vi "运维调试_质控单元.vi"() -> ()   [LabVIEW 2016, in "质控单元.lvlib"]
uses:
  <vilib>/Utility/miscctls.llb/LVPointTypeDef.ctl
  <vilib>/Analysis/6fits.llb/Curve Fitting Criteria.ctl
  <vilib>/Plasmionique/MB Master/MB_Master_Serial/MB_Master_Serial.lvclass
  D:/Program Files (x86)/National Instruments/LabVIEW 2016/vi.lib/Plasmionique/MB Master/MB_Master/MB_Master.lvclass
  <vilib>/Utility/config.llb/Read Key (I32).vi
  <vilib>/Utility/config.llb/Read Key (Double).vi
  <vilib>/Utility/config.llb/Read Key (Boolean).vi
  <vilib>/Utility/config.llb/Read Key (U32).vi
  <vilib>/Utility/config.llb/Write Key (I32).vi
  <vilib>/Utility/config.llb/Write Key (Double).vi
  <vilib>/Utility/config.llb/Write Key (Boolean).vi
  <vilib>/Utility/config.llb/Write Key (U32).vi
  <vilib>/Plasmionique/MB Master/MB Master.lvlib
  <vilib>/ptbypt/NI_PtbyPt.lvlib
  <vilib>/Utility/config.llb/NI_LVConfig.lvlib
  <vilib>/Analysis/NI_AALPro.lvlib
panel:
  in  "柱塞泵4":bool
  in  "CODCr量程选择":enum32{"H", "L", "AUTO"}(ring)
  in  "B 4":dbl caption="B4"
  in  "K 4":dbl caption="K4"
  out "通讯指示灯4":bool
  in  "CODCr选择":bool
  out "CODCr传感器故障报警":bool
  out "CODCr超时报警":bool
  out "CODMn超时报警":bool
  out "总磷总氮超时报警":bool
  out "氨氮进样超时报警":bool
  out "CODMn传感器故障报警":bool
  out "总磷总氮传感器故障报警":bool
  out "氨氮传感器故障报警":bool
  in  "CODCr加标回收启动":bool
  in  "CODCr停止":bool
  in  "CODCr排液":bool
  in  "CODCr调试":bool
  out "CODCr加标回收率":dbl caption="加标回收率" format="%.2f"
  out "CODCr加标体积":dbl caption="加标体积" format="%.3f"
  out "CODCr母液浓度":dbl caption="加标母液浓度" format="%.2f"
  out "CODCr加标水杯定容体积":dbl caption="加标水杯定容体积" format="%.2f"
  out "CODCr加标后水样浓度":dbl caption="加标后水样浓度" format="%.2f"
  out "CODCr加标前水样浓度":dbl caption="加标前水样浓度" format="%.2f"
  out "CODCr检出限":dbl caption="检出限" format="%.2f"
  out "CODCr量程":dbl caption="量程" format="%.2f"
  out "CODCr状态":u16(ring) caption="状态" items=["待机", "润洗", "进样", "等待取液", "排液"]
  out "质控流程中":bool
  out "CODMn质控中断报警":bool
  out "总磷质控中断报警":bool
  out "总氮质控中断报警":bool
  out "氨氮质控中断报警":bool
  in  "报警清除":bool
  in  "CODMn量程选择":enum32{"H", "L", "AUTO"}(ring)
  in  "CODMn加标回收启动":bool
  in  "总磷总氮加标回收启动":bool
  in  "氨氮加标回收启动":bool
  in  "总磷量程选择":enum32{"H", "L", "AUTO"}(ring)=enum."AUTO"
  in  "总氮量程选择":enum32{"H", "L", "AUTO"}(ring)=enum."AUTO"
  in  "氨氮量程选择":enum32{"H", "L", "AUTO"}(ring)=enum."AUTO"
  out "线性值":T1
  out "通讯指示灯3":bool
  out "通讯指示灯2":bool
  out "通讯指示灯1":bool
  in  "CODMn选择":bool
  in  "总氮模块选择":bool
  in  "氨氮、总磷模块":bool
  in  "枚举":enum16{"柱塞泵1", "柱塞泵2", "柱塞泵3", "柱塞泵4"}(ring)
  in  "启用":bool
  in  "B 3":dbl caption="B3"
  in  "K 3":dbl caption="K3"
  in  "B 2":dbl caption="B2"
  in  "K 2":dbl caption="K2"
  in  "B":dbl caption="B1"
  in  "K":dbl caption="K1"
  out "r^2":dbl format="%_6g"
  out "拟合方程":string
  in  "实际体积 5":dbl
  in  "标准体积 5":dbl
  in  "实际体积 4":dbl
  in  "标准体积 4":dbl
  in  "实际体积 3":dbl
  in  "实际体积 2":dbl
  in  "实际体积 1":dbl
  in  "标准体积 3":dbl
  in  "标准体积 2":dbl
  in  "标准体积 1":dbl
  in  "读取":bool
  in  "柱塞泵3":bool
  in  "柱塞泵2":bool
  in  "柱塞泵1":bool
  in  "注出体积选择":u16(ring) items=["0.1mL", "0.3mL", "0.5mL", "0.8mL", "1.0mL"]
  out "Serial Config":T2={"baud rate (bps)"=115200, "stop bits"=10, "parity"=0, "flow control"=0, "timeout"=100, "retries"=1} {"stop bits" items=["1.0"=10, "1.5"=15, "2.0"=20]; "parity" items=["None", "Odd", "Even", "Mark", "Space"]; "flow control" items=["None", "XON/XOFF", "RTS/CTS", "XON/XOFF & RTS/CTS", "DTR/DSR", "XON/XOFF & DTR/DSR"]}
  out "VISA Resource":refnum<visa-resource-name>="COM8"
  in  "背隙补偿步数 3":i32 min=0 max=2000
  in  "背隙补偿步数 2":i32 min=0 max=2000
  in  "写入":bool
  in  "背隙补偿步数":i32 min=0 max=2000
  out "启动模块":T3
  in  "总氮停止":bool
  in  "总氮排液":bool
  in  "总氮调试":bool
  out "总氮加标回收率":dbl caption="加标回收率" format="%.2f"
  out "总氮加标体积":dbl caption="加标体积" format="%.3f"
  out "总氮母液浓度":dbl caption="加标母液浓度" format="%.3f"
  out "总氮加标水杯定容体积":dbl caption="加标水杯定容体积" format="%.2f"
  out "总氮加标后水样浓度":dbl caption="加标后水样浓度" format="%.3f"
  out "总氮加标前水样浓度":dbl caption="加标前水样浓度" format="%.3f"
  out "总氮检出限":dbl caption="检出限" format="%.3f"
  out "总氮量程":dbl caption="量程" format="%.2f"
  out "总氮状态":u16(ring) caption="状态" items=["待机", "润洗", "进样", "等待取液", "排液"]
  in  "返回":bool
  in  "查看":bool
  out "直接启动":bool
  out "常规启动":bool
  out "columns":string[](array[string])
  out "data":T4
  out "COD平行样测完标志":bool
  out "氨氮总磷平行样测完标志":bool
  out "输出簇 2":T5
  out "常规启动 2":bool
  out "直接启动 2":bool
  out "启动模块 2":cluster{"氨氮1":bool, "总磷1":bool, " COD1":bool}
  in  "停止测量":bool
  out "输出簇":T6
  in  "加标回收":bool
  in  "平行样测试":bool
  in  "CODMn停止":bool
  in  "CODMn排液":bool
  in  "CODMn调试":bool
  in  "总磷停止":bool
  in  "总磷排液":bool
  in  "总磷调试":bool
  out "COD加标回收率":dbl caption="加标回收率" format="%.2f"
  out "COD加标体积":dbl caption="加标体积" format="%.3f"
  out "COD母液浓度":dbl caption="加标母液浓度" format="%.2f"
  out "COD加标水杯定容体积":dbl caption="加标水杯定容体积" format="%.2f"
  out "COD加标后水样浓度":dbl caption="加标后水样浓度" format="%.2f"
  out "COD加标前水样浓度":dbl caption="加标前水样浓度" format="%.2f"
  out "COD检出限":dbl caption="检出限" format="%.2f"
  out "COD量程":dbl caption="量程" format="%.2f"
  out "CODMn状态":u16(ring) caption="状态" items=["待机", "润洗", "进样", "等待取液", "排液"]
  out "总磷加标回收率":dbl caption="加标回收率" format="%.2f"
  out "总磷加标体积":dbl caption="加标体积" format="%.3f"
  out "总磷母液浓度":dbl caption="加标母液浓度" format="%.3f"
  out "总磷加标水杯定容体积":dbl caption="加标水杯定容体积" format="%.2f"
  out "总磷加标后水样浓度":dbl caption="加标后水样浓度" format="%.3f"
  out "总磷加标前水样浓度":dbl caption="加标前水样浓度" format="%.3f"
  out "总磷检出限":dbl caption="检出限" format="%.3f"
  out "总磷量程":dbl caption="量程" format="%.2f"
  out "总磷状态":u16(ring) caption="状态" items=["待机", "润洗", "进样", "等待取液", "排液"]
  out "氨氮加标回收率":dbl caption="加标回收率" format="%.2f"
  out "氨氮加标体积":dbl caption="加标体积" format="%.3f"
  out "氨氮母液浓度":dbl caption="加标母液浓度" format="%.3f"
  out "氨氮加标水杯定容体积":dbl caption="加标水杯定容体积" format="%.2f"
  out "氨氮加标后水样浓度":dbl caption="加标后水样浓度" format="%.3f"
  out "氨氮加标前水样浓度":dbl caption="加标前水样浓度" format="%.3f"
  out "氨氮检出限":dbl caption="检出限" format="%.3f"
  out "氨氮量程":dbl caption="量程" format="%.2f"
  out "氨氮状态":u16(ring) caption="状态" items=["待机", "润洗", "进样", "等待取液", "排液"]
  in  "氨氮停止":bool
  in  "氨氮排液":bool
  in  "氨氮调试":bool
  # "状态显示区"
  # "参数配置区"
  # "2000步等于1mL\n100步等于0.05mL\n20步等于0.01mL\n2步等于0.001mL\n（初始默认100步）"
  # "辅助计算区"
  # "柱塞泵调试区"
  # "CODCr质控参数"
  # "%"
  # "mL"
  # "mg/L"
  # "mL"
  # "mg/L"
  # "mg/L"
  # "mg/L"
  # "mg/L"
  # "总氮质控参数"
  # "%"
  # "mL"
  # "mg/L"
  # "mL"
  # "mg/L"
  # "mg/L"
  # "mg/L"
  # "mg/L"
  # "CODMn质控参数"
  # "%"
  # "mL"
  # "mg/L"
  # "mL"
  # "mg/L"
  # "mg/L"
  # "mg/L"
  # "mg/L"
  # "总磷质控参数"
  # "%"
  # "mL"
  # "mg/L"
  # "mL"
  # "mg/L"
  # "mg/L"
  # "mg/L"
  # "mg/L"
  # "氨氮质控参数"
  # "%"
  # "mL"
  # "mg/L"
  # "mL"
  # "mg/L"
  # "mg/L"
  # "mg/L"
  # "mg/L"
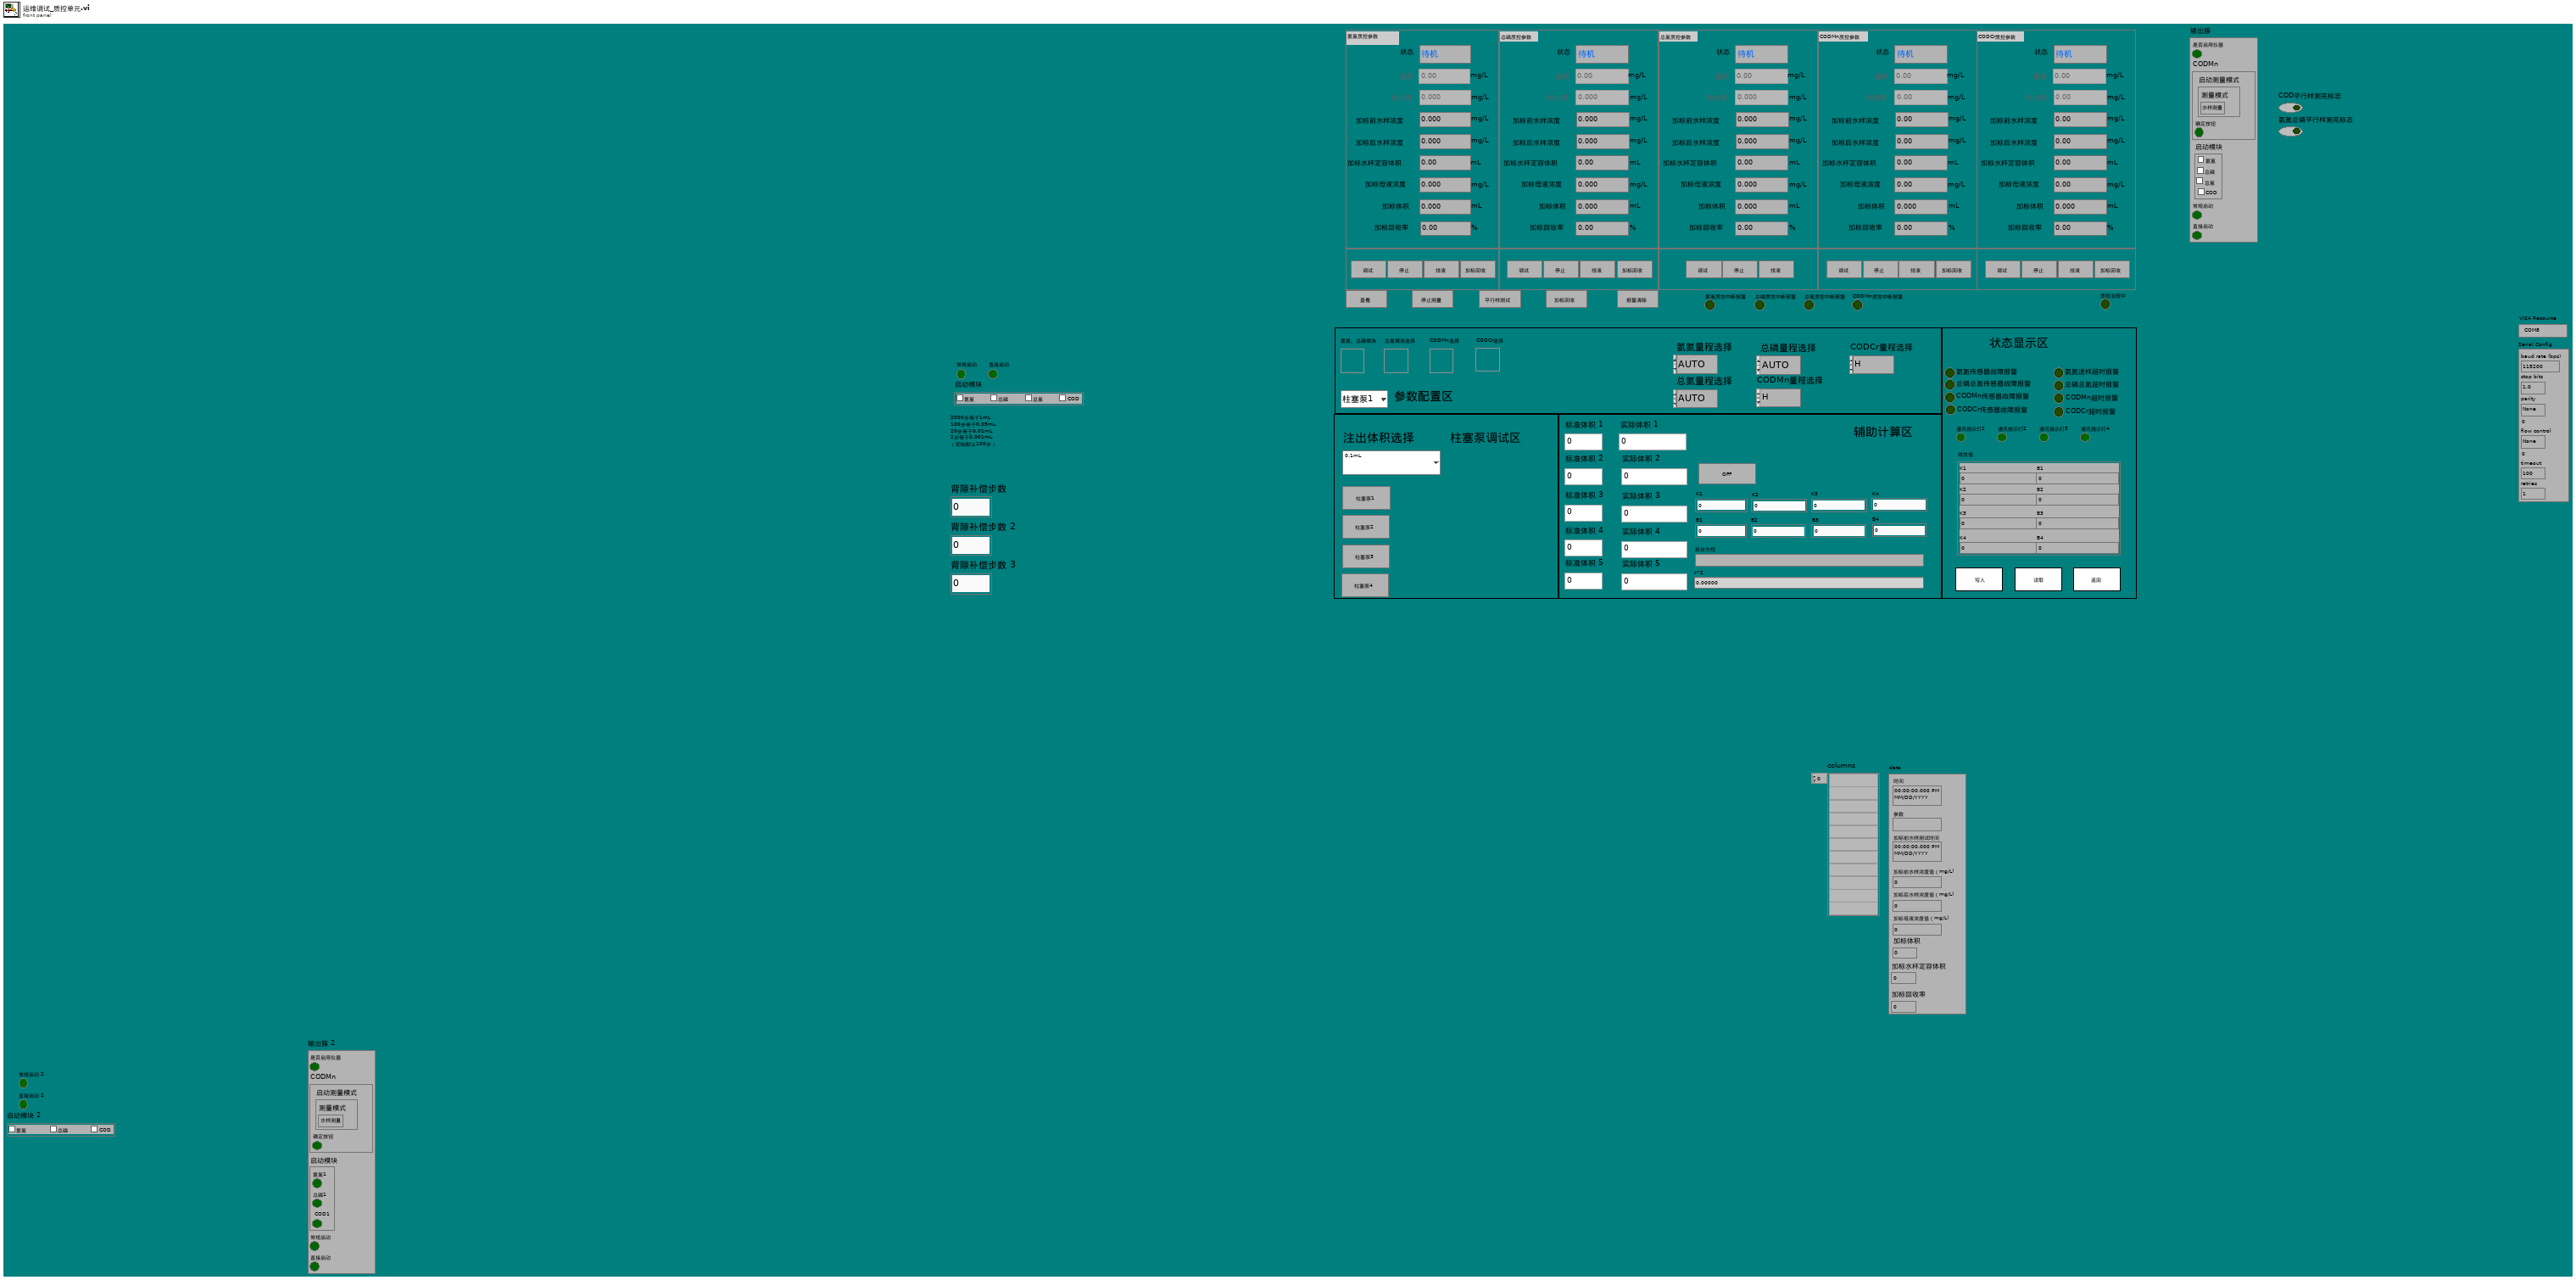
[diagram p1: front panel]
types:
  T1 = cluster{"K1":sgl, "B1":sgl, "K2":sgl, "B2":sgl, "K3":sgl, "B3":sgl, "K4":sgl, "B4":sgl}
  T2 = cluster{"baud rate (bps)":u32, "stop bits":u16, "parity":u16, "flow control":u16, "timeout":u32, "retries":i32}
  T3 = cluster{"氨氮":bool, "总磷":bool, "总氮":bool, "COD":bool}
  T4 = cluster{"时间":timestamp, "参数":string, "加标前水样测试时间":timestamp, "加标前水样浓度值（mg/L)":sgl, "加标后水样浓度值（mg/L)":sgl, "加标母液浓度值（mg/L)":sgl, "加标体积":dbl, "加标水杯定容体积":dbl, "加标回收率":dbl}
  T5 = cluster{"是否启用仪器":bool, "CODMn":cluster{"启动测量模式":cluster{"测量模式":enum16{"水样测量", "标样核查", "加标回收", "平行样", "校零", "校标"}}, "确定按钮":bool}, "启动模块":cluster{"氨氮1":bool, "总磷1":bool, " COD1":bool}, "常规启动":bool, "直接启动":bool}
  T6 = cluster{"是否启用仪器":bool, "CODMn":cluster{"启动测量模式":cluster{"测量模式":enum16{"水样测量", "标样核查", "加标回收", "平行样", "校零", "校标"}}, "确定按钮":bool}, "启动模块 3":cluster{"氨氮":bool, "总磷":bool, "总氮":bool, "COD":bool}, "常规启动":bool, "直接启动":bool}
  T7 = typedef "LVPointTypeDef.ctl" = cluster{"Horizontal":i16, "Vertical":i16}
  T8 = cluster{"量程":dbl, "检出限":dbl, "加标前水样浓度":dbl, "加标后水样浓度":dbl, "加标水杯定容体积":dbl, "加标母液浓度":dbl, "加标体积":dbl, "加标回收率":dbl}
  T9 = cluster{"因子编码":u32, "单位":u16, "标样参考值":sgl, "水样数据时间":timestamp, "水样实测值":sgl, "水样数据标识":string, "标样数据时间":timestamp, "标样实测值":sgl, "标样数据标识":string, "空白数据时间":timestamp, "空白实测值":sgl, "空白数据标识":string, "零点核查数据时间":timestamp, "零点核查实测值":sgl, "零点核查数据标识":string, "跨度核查数据时间":timestamp, "跨度核查实测值":sgl, "跨度核查数据标识":string, "加标回收数据时间":timestamp, "加标回收实测值":sgl, "加标回收数据标识":string, "平行样数据时间":timestamp, "平行样实测值":sgl, "平行样数据标识":string, "F0":sgl, "F1":sgl, "F2":sgl, "F3":sgl, "F4":sgl, "F5":sgl, "F6":sgl, "F7":sgl, "温度":sgl, "湿度":sgl, "X值":sgl}
  T10 = cluster{"因子编码":u32, "单位":u16, "标样参考值":sgl, "水样数据时间":timestamp, "水样实测值":sgl, "水样数据标识":string, "标样数据时间":timestamp, "标样实测值":sgl, "标样数据标识":string, "空白数据时间":timestamp, "空白实测值":sgl, "空白数据标识":string, "零点核查数据时间":timestamp, "零点核查实测值":sgl, "零点核查数据标识":string, "跨度核查数据时间":timestamp, "跨度核查实测值":sgl, "跨度核查数据标识":string, "加标回收数据时间":timestamp, "加标回收实测值":sgl, "加标回收数据标识":string, "平行样数据时间":timestamp, "平行样实测值":sgl, "平行样数据标识":string}
  T11 = enum8{"Enabled", "Disabled", "Disabled and Grayed Out"}
  T12 = typedef "NI_AALPro.lvlib/Curve Fitting Criteria.ctl" = u16
  T13 = typedef "NI_LVConfig.lvlib/Config Data RefNum.ctl" = refnum<k1>
  T14 = cluster{"是否启用仪器":bool, "CODMn":cluster{"启动测量模式":cluster{"测量模式":enum16{"水样测量", "标样核查", "加标回收", "平行样", "校零", "校标"}}, "确定按钮":bool}, "启动模块":cluster{"氨氮":bool, "总磷":bool, "总氮":bool, "COD":bool}, "常规启动":bool, "直接启动":bool}
  T15 = cluster{"命令":string, cluster{"starting address":u16, "holding register value":u16}}
  T16 = enum32{"Bad", "Idle", "Run top level", "Running"}
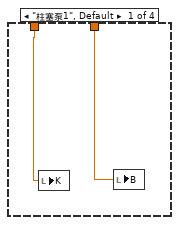
[diagram p3: hidden frame]
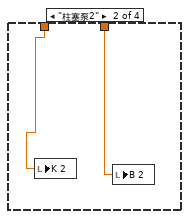
[diagram p4: hidden frame]
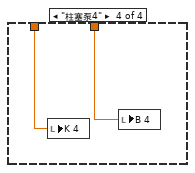
[diagram p5: hidden frame]
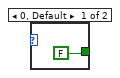
[diagram p8: hidden frame]
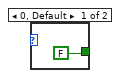
[diagram p9: hidden frame]
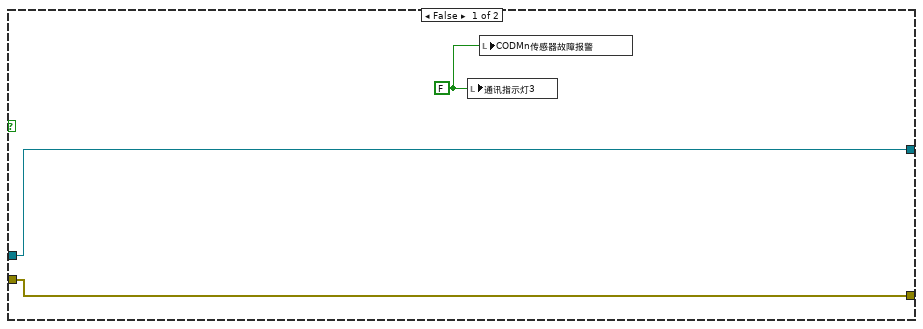
[diagram p10: hidden frame]
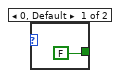
[diagram p11: hidden frame]
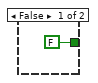
[diagram p12: hidden frame]
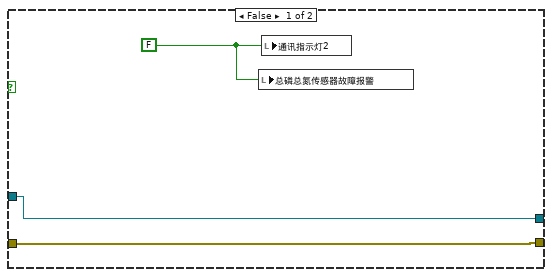
[diagram p13: hidden frame]
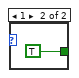
[diagram p14: hidden frame]
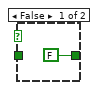
[diagram p15: hidden frame]
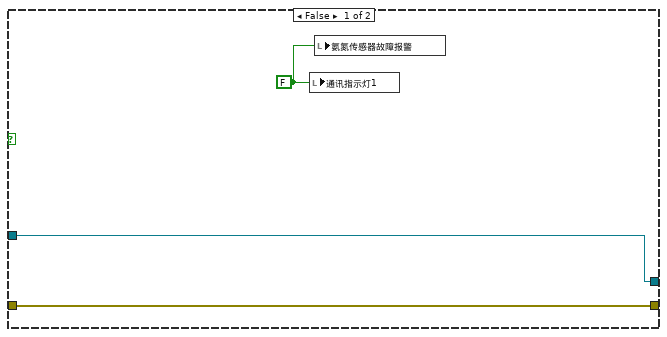
[diagram p16: hidden frame]
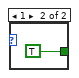
[diagram p17: hidden frame]
diagram:
  w21 = T2 {"baud rate (bps)"=115200, "stop bits"=10, "parity"=0, "flow control"=0, "timeout"=500, "retries"=1} ("Serial Config")
  w22 = refnum<visa-resource-name> "COM8" ("VISA Resource")
  n1 = global write "串口参数全局.vi" "Serial Config"(w21) -> ()
  n2 = control-ref of="总氮加标回收率"() -> (w36:refnum<vi>)
  n3 = control-ref of="总氮加标体积"() -> (w37:refnum<vi>)
  n4 = control-ref of="总氮加标水杯定容体积"() -> (w39:refnum<vi>)
  n5 = control-ref of="总氮加标后水样浓度"() -> (w40:refnum<vi>)
  n6 = control-ref of="总氮母液浓度"() -> (w38:refnum<vi>)
  n7 = global write "串口参数全局.vi" "VISA Resource"(w22) -> ()
  n8 = control-ref of="总氮检出限"() -> (w42:refnum<vi>)
  n9 = control-ref of="总氮加标前水样浓度"() -> (w41:refnum<vi>)
  n10 = control-ref of="总氮量程"() -> (w43:refnum<vi>)
  n11 = call <vilib>:"Open Serial Session.vi"("Mode (RTU)"=enum16{"RTU", "ASCII"}."RTU", "Slave ID"=u8 10, "Serial Config"=w21, "VISA Resource"=w22) -> ("Error out"=w54:errorcluster, "MB_Serial session"=w55:refnum<class "MB_Master_Serial.lvclass">)  [unwired: 6 in]
  n12 = control-ref of="COD加标水杯定容体积"() -> (w60:refnum<vi>)
  n13 = control-ref of="COD加标前水样浓度"() -> (w62:refnum<vi>)
  n14 = control-ref of="COD加标后水样浓度"() -> (w61:refnum<vi>)
  n15 = property on="窗格" class="Pane"("Origin"=T7 {"Horizontal"=0, "Vertical"=0} ("原点")) -> ()  [unwired: 2 in, 2 out]
  n16 = property on="窗格" class="Pane"("Origin"=T7 {"Horizontal"=0, "Vertical"=0} ("原点")) -> ()  [unwired: 2 in, 2 out]
  n17 = call "质控参数读取.vi"("section"="氨氮质控参数") -> ("error out"=w85:errorcluster, "参数"=w104:T8)  [unwired: 9 in]
  n18 = while {
    tunnel: w55 -> [w162]
    tunnel: w54 -> [w161]
    tunnel: [w128] -> w53
    tunnel: [w129] -> w23
    stop <- FALSE stop-if-true
    n19 = local read "氨氮、总磷模块"() -> (w135:bool)
    n20 = case shown="真" w135 {
      tunnel: w162 -> [w262 w282]
      tunnel: w161 -> [w261 w281]
      tunnel: [w262 w270] -> w139
      tunnel: [w261 w269] -> w137
      frame False {
        w260 = FALSE ("通讯指示灯1")
        n21 = local write "通讯指示灯1"(w260) -> ()
        n22 = local write "氨氮传感器故障报警"(w260) -> ()
      }
      frame True {
        n23 = property class="MB_Master_Serial"(reference=w282, "Properties:Slave ID"=u8 1 ("Slave ID")) -> (reference out=w277:refnum<class "MB_Master_Serial.lvclass">)  [unwired: 1 in, 1 out]
        n24 = call <vilib>:"Read Holding Registers.vi"("error in (no error)"=w281, "quantity"=u16 5, "starting address"=u16 100, "MB session in"=w277) -> ("error out"=w269:errorcluster, "Registers"=w278:u16[], "MB session out"=w270:refnum<class "MB_Master_Serial.lvclass">)  [unwired: 5 in]
        n25 = Index Array(array=w278, index #2=4 ("索引"), index #3=5 ("索引")) -> (element #1=w263:u16, element #2=w274:u16, element #3=w265:u16)  [unwired: 1 in]
        "氨氮状态" <- w263
        n26 = Unbundle By Name(w269) -> ("status"=w268:bool)
        n27 = case shown="0, 默认" w265 {
          tunnel: [FALSE TRUE] -> w264
          frame 0, Default {
          }
          frame 1 {
          }
        }
        "氨氮进样超时报警" <- w264
        n28 = global write "氨氮加标回收状态全局变量.vi" "氨氮状态"(w263) -> ()
        n29 = Not(x=w268) -> (.not. x?=→"通讯指示灯1":bool)
        n30 = Equal?(x=w274, y=u16 1) -> (x = y?=w271:bool)
        n31 = case shown="假" w271 {
          tunnel: w271 -> [_ w286]
          tunnel: [FALSE w286] -> w272
          frame False {
          }
          frame True {
          }
        }
        "氨氮传感器故障报警" <- w272
      }
    }
    n32 = local read "CODCr加标前水样浓度"() -> (w126:dbl)
    n33 = global read "水样浓度全局.vi" "CODCr加标前水样浓度"() -> (w127:dbl)
    n34 = global read "质控测完标志全局 1.vi" "总磷总氮平行样测完标志"() -> (→"氨氮总磷平行样测完标志":bool)
    n35 = global read "质控测完标志全局 1.vi" "氨氮加标回收测完标志"() -> (w148:bool)
    n36 = global read "质控测完标志全局 1.vi" "总磷加标回收测完标志"() -> (w140:bool)
    n37 = global read "质控测完标志全局 1.vi" "COD平行样测完标志"() -> (→"COD平行样测完标志":bool)
    n38 = global read "水样浓度全局.vi" "COD加标前水样浓度"() -> (w156:dbl)
    n39 = local read "总氮加标前水样浓度"() -> (w143:dbl)
    n40 = global read "水样浓度全局.vi" "氨氮加标前水样浓度"() -> (w160:dbl)
    n41 = global read "水样浓度全局.vi" "总磷加标前水样浓度"() -> (w158:dbl)
    n42 = local read "COD加标前水样浓度"() -> (w155:dbl)
    n43 = global read "水样浓度全局.vi" "总氮加标前水样浓度"() -> (w142:dbl)
    n44 = local read "氨氮加标前水样浓度"() -> (w159:dbl)
    n45 = local read "总磷加标前水样浓度"() -> (w157:dbl)
    n46 = global read "质控测完标志全局 1.vi" "COD加标回收测完标志"() -> (w123:bool)
    n47 = global read "质控测完标志全局 1.vi" "CODCr加标回收测完标志"() -> (w117:bool)
    n48 = global read "质控测完标志全局 1.vi" "总氮加标回收测完标志"() -> (w120:bool)
    n49 = Wait (ms)(milliseconds to wait=u32 1000 ("等待时间（毫秒）")) -> ()  [unwired: 1 out]
    n50 = Not Equal?(x=w127, y=w126) -> (x != y?=w125:bool)
    n51 = Not Equal?(x=w160, y=w159) -> (x != y?=w154:bool)
    n52 = Not Equal?(x=w158, y=w157) -> (x != y?=w152:bool)
    n53 = Not Equal?(x=w156, y=w155) -> (x != y?=w151:bool)
    n54 = Not Equal?(x=w142, y=w143) -> (x != y?=w141:bool)
    n55 = call <vilib>:"Boolean Crossing PtByPt.vi"("direction"=enum16{"either", "false-true", "true-false"}."false-true", "input"=w148) -> ("crossing"=w147:bool)  [unwired: 1 in]
    n56 = call <vilib>:"Boolean Crossing PtByPt.vi"("direction"=enum16{"either", "false-true", "true-false"}."false-true", "input"=w140) -> ("crossing"=w144:bool)  [unwired: 1 in]
    n57 = call <vilib>:"Boolean Crossing PtByPt.vi"("direction"=enum16{"either", "false-true", "true-false"}."false-true", "input"=w123) -> ("crossing"=w122:bool)  [unwired: 1 in]
    n58 = call <vilib>:"Boolean Crossing PtByPt.vi"("direction"=enum16{"either", "false-true", "true-false"}."false-true", "input"=w120) -> ("crossing"=w119:bool)  [unwired: 1 in]
    n59 = call <vilib>:"Boolean Crossing PtByPt.vi"("direction"=enum16{"either", "false-true", "true-false"}."false-true", "input"=w117) -> ("crossing"=w116:bool)  [unwired: 1 in]
    n60 = case shown="真" w147 {
      frame False {
      }
      frame True {
        n61 = flat-sequence {
          frame #0 {
            n62 = global read "VAR氨氮全局变量.vi" "测量数据区"() -> (w338:T9)
            n63 = Unbundle By Name(w338) -> ("加标回收实测值"=w339:sgl)
            n64 = property on="氨氮加标后水样浓度" class="DigNum (严格)"("Val(Sgnl)"=w339) -> ()  [unwired: 2 in, 2 out]
          }
          frame #1 {
            n65 = Wait (ms)(milliseconds to wait=u32 500 ("等待时间（毫秒）")) -> ()  [unwired: 1 out]
          }
          frame #2 {
            n66 = global read "VAR氨氮全局变量.vi" "测量数据区"() -> (w344:T9)
            n67 = local read "氨氮加标水杯定容体积"() -> (w350:dbl)
            n68 = global read "水样浓度全局.vi" "氨氮加标前水样浓度"() -> (w354:dbl)
            n69 = Unbundle By Name(w344) -> ("加标回收数据时间"=w347:timestamp)
            n70 = Unbundle By Name(w344) -> ("加标回收实测值"=w353:sgl)
            n71 = Unbundle By Name(w344) -> ("水样数据时间"=w345:timestamp)
            n72 = local read "氨氮加标回收率"() -> (w349:dbl)
            n73 = local read "氨氮母液浓度"() -> (w352:dbl)
            n74 = local read "氨氮加标体积"() -> (w351:dbl)
            n75 = Bundle By Name(cluster=T4 {"时间"=timestamp(0 s since 1904-01-01), "参数"="", "加标前水样测试时间"=timestamp(0 s since 1904-01-01), "加标前水样浓度值（mg/L)"=0.0, "加标后水样浓度值（mg/L)"=0.0, "加标母液浓度值（mg/L)"=0.0, "加标体积"=0.0, "加标水杯定容体积"=0.0, "加标回收率"=0.0} ("data"), "时间"=w347, "参数"="氨氮加标回收率" ("table"), "加标前水样测试时间"=w345, "加标前水样浓度值（mg/L)"=w354, "加标后水样浓度值（mg/L)"=w353, "加标母液浓度值（mg/L)"=w352, "加标体积"=w351, "加标水杯定容体积"=w350, "加标回收率"=w349) -> (w341:T4)
            n76 = local read "columns"() -> (w342:string[])
            n77 = local write "data"(w341) -> ()
            n78 = call "数据写入databaseZK.vi"("data"=w341, "columns"=w342, "table"="加标回收率") -> ()  [unwired: 8 in, 1 out]
          }
        }
      }
    }
    n79 = case shown="真" w144 {
      frame False {
      }
      frame True {
        n80 = flat-sequence {
          frame #0 {
            n81 = global read "VAR总磷总氮全局变量.vi" "总磷测量数据区"() -> (w321:T9)
            n82 = Unbundle By Name(w321) -> ("加标回收实测值"=w322:sgl)
            n83 = property on="总磷加标后水样浓度" class="DigNum (严格)"("Val(Sgnl)"=w322) -> ()  [unwired: 2 in, 2 out]
          }
          frame #1 {
            n84 = Wait (ms)(milliseconds to wait=u32 500 ("等待时间（毫秒）")) -> ()  [unwired: 1 out]
          }
          frame #2 {
            n85 = global read "VAR总磷总氮全局变量.vi" "总磷测量数据区"() -> (w327:T9)
            n86 = Unbundle By Name(w327) -> ("加标回收数据时间"=w330:timestamp)
            n87 = Unbundle By Name(w327) -> ("加标回收实测值"=w328:sgl)
            n88 = Unbundle By Name(w327) -> ("水样数据时间"=w329:timestamp)
            n89 = local read "总磷加标水杯定容体积"() -> (w334:dbl)
            n90 = local read "总磷加标回收率"() -> (w333:dbl)
            n91 = local read "总磷母液浓度"() -> (w336:dbl)
            n92 = local read "总磷加标体积"() -> (w335:dbl)
            n93 = global read "水样浓度全局.vi" "总磷加标前水样浓度"() -> (w337:dbl)
            n94 = Bundle By Name(cluster=T4 {"时间"=timestamp(0 s since 1904-01-01), "参数"="", "加标前水样测试时间"=timestamp(0 s since 1904-01-01), "加标前水样浓度值（mg/L)"=0.0, "加标后水样浓度值（mg/L)"=0.0, "加标母液浓度值（mg/L)"=0.0, "加标体积"=0.0, "加标水杯定容体积"=0.0, "加标回收率"=0.0} ("data"), "时间"=w330, "参数"="总磷加标回收率" ("table"), "加标前水样测试时间"=w329, "加标前水样浓度值（mg/L)"=w337, "加标后水样浓度值（mg/L)"=w328, "加标母液浓度值（mg/L)"=w336, "加标体积"=w335, "加标水杯定容体积"=w334, "加标回收率"=w333) -> (w324:T4)
            "data" <- w324
            n95 = local read "columns"() -> (w325:string[])
            n96 = call "数据写入databaseZK.vi"("data"=w324, "columns"=w325, "table"="加标回收率") -> ()  [unwired: 8 in, 1 out]
          }
        }
      }
    }
    n97 = case shown="真" w122 {
      frame False {
      }
      frame True {
        n98 = flat-sequence {
          frame #0 {
            n99 = global read "COD浓度全局变量.vi" "COD浓度（mg/L)"() -> (w306:dbl)
            n100 = property on="COD加标后水样浓度" class="DigNum (严格)"("Val(Sgnl)"=w306) -> ()  [unwired: 2 in, 2 out]
          }
          frame #1 {
            n101 = Wait (ms)(milliseconds to wait=u32 500 ("等待时间（毫秒）")) -> ()  [unwired: 1 out]
          }
          frame #2 {
            n102 = local read "COD加标水杯定容体积"() -> (w316:dbl)
            n103 = global read "水样浓度全局.vi" "COD加标前水样浓度"() -> (w320:dbl)
            n104 = global read "COD浓度全局变量.vi" "COD浓度（mg/L)"() -> (w319:dbl)
            n105 = global read "COD测量模式全局.vi" "加标回收启动时间"() -> (w312:timestamp)
            n106 = global read "COD测量模式全局.vi" "水样启动时间"() -> (w311:timestamp)
            n107 = local read "COD加标回收率"() -> (w315:dbl)
            n108 = local read "COD母液浓度"() -> (w318:dbl)
            n109 = local read "COD加标体积"() -> (w317:dbl)
            n110 = Bundle By Name(cluster=T4 {"时间"=timestamp(0 s since 1904-01-01), "参数"="", "加标前水样测试时间"=timestamp(0 s since 1904-01-01), "加标前水样浓度值（mg/L)"=0.0, "加标后水样浓度值（mg/L)"=0.0, "加标母液浓度值（mg/L)"=0.0, "加标体积"=0.0, "加标水杯定容体积"=0.0, "加标回收率"=0.0} ("data"), "时间"=w312, "参数"="CODMn加标回收率" ("table"), "加标前水样测试时间"=w311, "加标前水样浓度值（mg/L)"=w320, "加标后水样浓度值（mg/L)"=w319, "加标母液浓度值（mg/L)"=w318, "加标体积"=w317, "加标水杯定容体积"=w316, "加标回收率"=w315) -> (w308:T4)
            n111 = local read "columns"() -> (w309:string[])
            n112 = local write "data"(w308) -> ()
            n113 = call "数据写入databaseZK.vi"("data"=w308, "columns"=w309, "table"="加标回收率") -> ()  [unwired: 8 in, 1 out]
          }
        }
      }
    }
    n114 = case shown="真" w119 {
      frame False {
      }
      frame True {
        n115 = flat-sequence {
          frame #0 {
            n116 = global read "VAR总磷总氮全局变量.vi" "总氮测量数据区"() -> (w288:T9)
            n117 = Unbundle By Name(w288) -> ("加标回收实测值"=w287:sgl)
            n118 = property on="总氮加标后水样浓度" class="DigNum (严格)"("Val(Sgnl)"=w287) -> ()  [unwired: 2 in, 2 out]
          }
          frame #1 {
            n119 = Wait (ms)(milliseconds to wait=u32 500 ("等待时间（毫秒）")) -> ()  [unwired: 1 out]
          }
          frame #2 {
            n120 = global read "VAR总磷总氮全局变量.vi" "总氮测量数据区"() -> (w298:T9)
            n121 = global read "VAR总磷总氮全局变量.vi" "总氮测量数据区"() -> (w294:T9)
            n122 = global read "VAR总磷总氮全局变量.vi" "总氮测量数据区"() -> (w304:T9)
            n123 = local read "总氮加标水杯定容体积"() -> (w300:dbl)
            n124 = global read "水样浓度全局.vi" "总氮加标前水样浓度"() -> (w305:dbl)
            n125 = Unbundle By Name(w298) -> ("加标回收数据时间"=w295:timestamp)
            n126 = Unbundle By Name(w304) -> ("加标回收实测值"=w303:sgl)
            n127 = Unbundle By Name(w294) -> ("水样数据时间"=w293:timestamp)
            n128 = local read "总氮加标回收率"() -> (w299:dbl)
            n129 = local read "总氮母液浓度"() -> (w302:dbl)
            n130 = local read "总氮加标体积"() -> (w301:dbl)
            n131 = Bundle By Name(cluster=T4 {"时间"=timestamp(0 s since 1904-01-01), "参数"="", "加标前水样测试时间"=timestamp(0 s since 1904-01-01), "加标前水样浓度值（mg/L)"=0.0, "加标后水样浓度值（mg/L)"=0.0, "加标母液浓度值（mg/L)"=0.0, "加标体积"=0.0, "加标水杯定容体积"=0.0, "加标回收率"=0.0} ("data"), "时间"=w295, "参数"="总氮加标回收率" ("table"), "加标前水样测试时间"=w293, "加标前水样浓度值（mg/L)"=w305, "加标后水样浓度值（mg/L)"=w303, "加标母液浓度值（mg/L)"=w302, "加标体积"=w301, "加标水杯定容体积"=w300, "加标回收率"=w299) -> (w290:T4)
            n132 = local read "columns"() -> (w291:string[])
            n133 = local write "data"(w290) -> ()
            n134 = call "数据写入databaseZK.vi"("data"=w290, "columns"=w291, "table"="加标回收率") -> ()  [unwired: 8 in, 1 out]
          }
        }
      }
    }
    n135 = case shown="真" w116 {
      frame False {
      }
      frame True {
        n136 = flat-sequence {
          frame #0 {
            n137 = global read "CODcr全局变量.vi" "测量数据区"() -> (w166:T10)
            n138 = Unbundle By Name(w166) -> ("加标回收实测值"=w165:sgl)
            n139 = property on="CODCr加标后水样浓度" class="DigNum (严格)"("Val(Sgnl)"=w165) -> ()  [unwired: 2 in, 2 out]
          }
          frame #1 {
            n140 = Wait (ms)(milliseconds to wait=u32 500 ("等待时间（毫秒）")) -> ()  [unwired: 1 out]
          }
          frame #2 {
            n141 = global read "CODcr全局变量.vi" "测量数据区"() -> (w174:T10)
            n142 = global read "CODcr全局变量.vi" "测量数据区"() -> (w173:T10)
            n143 = global read "CODcr全局变量.vi" "测量数据区"() -> (w172:T10)
            n144 = local read "CODCr加标水杯定容体积"() -> (w169:dbl)
            n145 = local read "CODCr加标回收率"() -> (w168:dbl)
            n146 = local read "CODCr母液浓度"() -> (w171:dbl)
            n147 = local read "CODCr加标体积"() -> (w170:dbl)
            n148 = global read "水样浓度全局.vi" "CODCr加标前水样浓度"() -> (w183:dbl)
            n149 = Unbundle By Name(w172) -> ("加标回收数据时间"=w179:timestamp)
            n150 = Unbundle By Name(w174) -> ("加标回收实测值"=w182:sgl)
            n151 = Unbundle By Name(w173) -> ("水样数据时间"=w178:timestamp)
            n152 = Bundle By Name(cluster=T4 {"时间"=timestamp(0 s since 1904-01-01), "参数"="", "加标前水样测试时间"=timestamp(0 s since 1904-01-01), "加标前水样浓度值（mg/L)"=0.0, "加标后水样浓度值（mg/L)"=0.0, "加标母液浓度值（mg/L)"=0.0, "加标体积"=0.0, "加标水杯定容体积"=0.0, "加标回收率"=0.0} ("data"), "时间"=w179, "参数"="CODCr加标回收率" ("table"), "加标前水样测试时间"=w178, "加标前水样浓度值（mg/L)"=w183, "加标后水样浓度值（mg/L)"=w182, "加标母液浓度值（mg/L)"=w171, "加标体积"=w170, "加标水杯定容体积"=w169, "加标回收率"=w168) -> (w175:T4)
            n153 = local read "columns"() -> (w176:string[])
            n154 = local write "data"(w175) -> ()
            n155 = call "数据写入databaseZK.vi"("data"=w175, "columns"=w176, "table"="加标回收率") -> ()  [unwired: 8 in, 1 out]
          }
        }
      }
    }
    n156 = Compound Arithmetic op=OR ("复合运算")(w154, w152, w151, w141, w125) -> (w153:bool)
    n157 = case shown="真" w153 {
      frame False {
      }
      frame True {
        n158 = global read "水样浓度全局.vi" "CODCr加标前水样浓度"() -> (w355:dbl)
        n159 = property on="CODCr加标前水样浓度" class="DigNum (严格)"("Val(Sgnl)"=w355) -> ()  [unwired: 2 in, 2 out]
        n160 = global read "水样浓度全局.vi" "COD加标前水样浓度"() -> (w357:dbl)
        n161 = global read "水样浓度全局.vi" "总氮加标前水样浓度"() -> (w356:dbl)
        n162 = global read "水样浓度全局.vi" "总磷加标前水样浓度"() -> (w358:dbl)
        n163 = global read "水样浓度全局.vi" "氨氮加标前水样浓度"() -> (w359:dbl)
        n164 = property on="总氮加标前水样浓度" class="DigNum (严格)"("Val(Sgnl)"=w356) -> ()  [unwired: 2 in, 2 out]
        n165 = property on="COD加标前水样浓度" class="DigNum (严格)"("Val(Sgnl)"=w357) -> ()  [unwired: 2 in, 2 out]
        n166 = property on="总磷加标前水样浓度" class="DigNum (严格)"("Val(Sgnl)"=w358) -> ()  [unwired: 2 in, 2 out]
        n167 = property on="氨氮加标前水样浓度" class="DigNum (严格)"("Val(Sgnl)"=w359) -> ()  [unwired: 2 in, 2 out]
      }
    }
    n168 = local read "总氮模块选择"() -> (w134:bool)
    n169 = case shown="真" w134 {
      tunnel: w139 -> [w236 w250]
      tunnel: [w236 w249] -> w138
      tunnel: w137 -> [w235 w248]
      tunnel: [w235 w246] -> w136
      frame False {
        w234 = FALSE ("通讯指示灯2")
        n170 = local write "总磷总氮传感器故障报警"(w234) -> ()
        n171 = local write "通讯指示灯2"(w234) -> ()
      }
      frame True {
        n172 = property class="MB_Master_Serial"(reference=w250, "Properties:Slave ID"=u8 2 ("Slave ID")) -> (reference out=w252:refnum<class "MB_Master_Serial.lvclass">)  [unwired: 1 in, 1 out]
        n173 = call <vilib>:"Read Holding Registers.vi"("error in (no error)"=w248, "quantity"=u16 5, "starting address"=u16 100, "MB session in"=w252) -> ("error out"=w246:errorcluster, "Registers"=w255:u16[], "MB session out"=w249:refnum<class "MB_Master_Serial.lvclass">)  [unwired: 5 in]
        n174 = Unbundle By Name(w246) -> ("status"=w247:bool)
        n175 = Index Array(array=w255, index #2=4 ("索引")) -> (element #1=w239:u16, element #2=w242:u16, element #3=w237:u16)  [unwired: 2 in]
        "总氮状态" <- w239
        "总磷状态" <- w239
        n176 = case shown="0, 默认" w237 {
          tunnel: [FALSE TRUE] -> w238
          frame 0, Default {
          }
          frame 1 {
          }
        }
        "总磷总氮超时报警" <- w238
        n177 = Not(x=w247) -> (.not. x?=→"通讯指示灯2":bool)
        n178 = Equal?(x=w242, y=u16 1) -> (x = y?=w240:bool)
        n179 = case shown="真" w240 {
          tunnel: w240 -> [_ w259]
          tunnel: [FALSE w259] -> w241
          frame False {
          }
          frame True {
          }
        }
        "总磷总氮传感器故障报警" <- w241
        n180 = global write "氨氮加标回收状态全局变量.vi" "总磷状态"(w239) -> ()
        n181 = global write "氨氮加标回收状态全局变量.vi" "总氮状态"(w239) -> ()
      }
    }
    n182 = local read "CODMn选择"() -> (w133:bool)
    n183 = case shown="真" w133 {
      tunnel: [w210 w225] -> w130
      tunnel: w138 -> [w210 w217]
      tunnel: w136 -> [w209 w216]
      tunnel: [w209 w214] -> w131
      frame False {
        w208 = FALSE ("通讯指示灯3")
        n184 = local write "通讯指示灯3"(w208) -> ()
        n185 = local write "CODMn传感器故障报警"(w208) -> ()
      }
      frame True {
        n186 = property class="MB_Master_Serial"(reference=w217, "Properties:Slave ID"=u8 3 ("Slave ID")) -> (reference out=w228:refnum<class "MB_Master_Serial.lvclass">)  [unwired: 1 in, 1 out]
        n187 = call <vilib>:"Read Holding Registers.vi"("error in (no error)"=w216, "quantity"=u16 5, "starting address"=u16 100, "MB session in"=w228) -> ("error out"=w214:errorcluster, "Registers"=w224:u16[], "MB session out"=w225:refnum<class "MB_Master_Serial.lvclass">)  [unwired: 5 in]
        n188 = Unbundle By Name(w214) -> ("status"=w215:bool)
        n189 = Index Array(array=w224, index #2=4 ("索引")) -> (element #1=w222:u16, element #2=w219:u16, element #3=w211:u16)  [unwired: 2 in]
        "CODMn状态" <- w222
        n190 = global write "氨氮加标回收状态全局变量.vi" "COD状态"(w222) -> ()
        n191 = Not(x=w215) -> (.not. x?=→"通讯指示灯3":bool)
        n192 = case shown="1" w211 {
          tunnel: [FALSE TRUE] -> w212
          frame 0, Default {
          }
          frame 1 {
          }
        }
        "CODMn超时报警" <- w212
        n193 = Equal?(x=w219, y=u16 1) -> (x = y?=w221:bool)
        n194 = case shown="真" w221 {
          tunnel: w221 -> [_ w233]
          tunnel: [FALSE w233] -> w218
          frame False {
          }
          frame True {
          }
        }
        "CODMn传感器故障报警" <- w218
      }
    }
    n195 = local read "CODCr选择"() -> (w132:bool)
    n196 = case shown="真" w132 {
      tunnel: w131 -> [w184 w202]
      tunnel: w130 -> [w185 w201]
      tunnel: [w185 w194] -> w129
      tunnel: [w184 w193] -> w128
      frame False {
      }
      frame True {
        n197 = property class="MB_Master_Serial"(reference=w201, error in=w202, "Properties:Slave ID"=u8 4 ("Slave ID")) -> (reference out=w196:refnum<class "MB_Master_Serial.lvclass">, error out=w195:errorcluster)
        n198 = call <vilib>:"Read Holding Registers.vi"("error in (no error)"=w195, "quantity"=u16 5, "starting address"=u16 100, "MB session in"=w196) -> ("error out"=w193:errorcluster, "Registers"=w198:u16[], "MB session out"=w194:refnum<class "MB_Master_Serial.lvclass">)  [unwired: 5 in]
        n199 = Unbundle By Name(w193) -> ("status"=w192:bool)
        n200 = Index Array(array=w198, index #2=4 ("索引")) -> (element #1=w190:u16, element #2=w187:u16, element #3=w189:u16)  [unwired: 2 in]
        "CODCr状态" <- w190
        n201 = global write "氨氮加标回收状态全局变量.vi" "CODCr状态"(w190) -> ()
        n202 = Not(x=w192) -> (.not. x?=→"通讯指示灯4":bool)
        n203 = case shown="1" w187 {
          tunnel: [FALSE TRUE] -> w186
          frame 0, Default {
          }
          frame 1 {
          }
        }
        "CODCr传感器故障报警" <- w186
        n204 = case shown="1" w189 {
          tunnel: [FALSE TRUE] -> w188
          frame 0, Default {
          }
          frame 1 {
          }
        }
        "CODCr超时报警" <- w188
      }
    }
  }
  n205 = Build Array(w43, w42, w41, w40, w39, w38, w37, w36) -> (w35:refnum<vi>[])
  n206 = while {
    stop <- FALSE stop-if-true
    n207 = global read "质控测完标志全局 1.vi" "氨氮质控流程中"() -> (w370:bool)
    n208 = global read "质控测完标志全局 1.vi" "COD质控流程中"() -> (w362:bool)
    n209 = global read "质控测完标志全局 1.vi" "总氮质控流程中"() -> (w366:bool)
    n210 = global read "质控中断报警全局.vi" "CODMn中断报警"() -> (→"CODMn质控中断报警":bool)
    n211 = global read "质控中断报警全局.vi" "氨氮中断报警"() -> (→"氨氮质控中断报警":bool)
    n212 = global read "质控中断报警全局.vi" "总氮中断报警"() -> (→"总氮质控中断报警":bool)
    n213 = Wait (ms)(milliseconds to wait=u32 100 ("等待时间（毫秒）")) -> ()  [unwired: 1 out]
    n214 = global read "质控中断报警全局.vi" "总磷中断报警"() -> (→"总磷质控中断报警":bool)
    n215 = local read "CODMn状态"() -> (w387:u16)
    n216 = global read "质控测完标志全局 1.vi" "质控流程中"() -> (w373:bool)
    "质控流程中" <- w373
    n217 = local read "总氮状态"() -> (w385:u16)
    n218 = local read "氨氮状态"() -> (w401:u16)
    n219 = local read "总磷状态"() -> (w392:u16)
    n220 = Not Equal To 0?(x=w385) -> (x != 0?=w384:bool)
    n221 = Not Equal To 0?(x=w401) -> (x != 0?=w400:bool)
    n222 = Not Equal To 0?(x=w392) -> (x != 0?=w394:bool)
    n223 = Not Equal To 0?(x=w387) -> (x != 0?=w391:bool)
    n224 = Select(t=T11."Disabled and Grayed Out" ("禁用"), s=w400, f=T11."Enabled") -> (s? t:f=w397:T11)
    n225 = Select(t=T11."Disabled and Grayed Out" ("禁用"), s=w394, f=T11."Enabled") -> (s? t:f=w393:T11)
    n226 = Select(t=T11."Disabled and Grayed Out" ("禁用"), s=w391, f=T11."Enabled") -> (s? t:f=w388:T11)
    n227 = Select(t=T11."Disabled and Grayed Out" ("禁用"), s=w370, f=T11."Enabled") -> (s? t:f=w368:T11)
    n228 = Select(t=T11."Disabled and Grayed Out" ("禁用"), s=w362, f=T11."Enabled") -> (s? t:f=w360:T11)
    n229 = Select(t=T11."Disabled and Grayed Out" ("禁用"), s=w366, f=T11."Enabled") -> (s? t:f=w364:T11)
    n230 = Select(t=T11."Disabled and Grayed Out" ("禁用"), s=w384, f=T11."Enabled") -> (s? t:f=w381:T11)
    n231 = Select(t=T11."Disabled and Grayed Out" ("禁用"), s=w373, f=T11."Enabled") -> (s? t:f=w372:T11)
    n232 = property on="氨氮加标回收启动" class="Bool"("DisabledEnum"=w368) -> ()  [unwired: 2 in, 2 out]
    n233 = property on="氨氮调试" class="Bool"("DisabledEnum"=w397) -> ()  [unwired: 2 in, 2 out]
    n234 = property on="总磷调试" class="Bool"("DisabledEnum"=w393) -> ()  [unwired: 2 in, 2 out]
    n235 = property on="COD调试" class="Bool"("DisabledEnum"=w388) -> ()  [unwired: 2 in, 2 out]
    n236 = property on="总磷总氮加标回收启动" class="Bool"("DisabledEnum"=w364) -> ()  [unwired: 2 in, 2 out]
    n237 = property on="CODMn加标回收启动" class="Bool"("DisabledEnum"=w360) -> ()  [unwired: 2 in, 2 out]
    n238 = property on="加标回收" class="Bool"("DisabledEnum"=w372) -> ()  [unwired: 2 in, 2 out]
    n239 = property on="总氮调试" class="Bool"("DisabledEnum"=w381) -> ()  [unwired: 2 in, 2 out]
    n240 = case shown="真" "启用" {
      frame False {
      }
      frame True {
        w419 = T12 0 items=["最小二乘", "最小绝对残差", "Bisquare"] ("method")
        n241 = Build Array("标准体积 1", "标准体积 2", "标准体积 3", "标准体积 4", "标准体积 5") -> (w416:dbl[])
        n242 = Build Array("实际体积 1", "实际体积 2", "实际体积 3", "实际体积 4", "实际体积 5") -> (w417:dbl[])
        n243 = call "线性公式质控用.vi"("标液浓度"=w416, "模型"=enum32{"线性", "多项式"}."线性", "监测浓度"=w417, "启用"=bool[] [TRUE, TRUE, TRUE, TRUE, TRUE], "method"=w419) -> ("拟合方程"=→"拟合方程":string, "r^2"=→"r^2":dbl, "slope"=w405:dbl, "intercept"=w404:dbl)  [unwired: 6 in, 1 out]
        n244 = case shown="\"柱塞泵3\"" "枚举" {
          tunnel: w405 -> [w423 w426 w427 w430]
          tunnel: w404 -> [w424 w425 w428 w429]
          frame "柱塞泵1", Default {
            n245 = local write "K"(w423) -> ()
            n246 = local write "B"(w424) -> ()
          }
          frame "柱塞泵2" {
            n247 = local write "K 2"(w426) -> ()
            n248 = local write "B 2"(w425) -> ()
          }
          frame "柱塞泵3" {
            n249 = local write "K 3"(w427) -> ()
            n250 = local write "B 3"(w428) -> ()
          }
          frame "柱塞泵4" {
            n251 = local write "K 4"(w430) -> ()
            n252 = local write "B 4"(w429) -> ()
          }
        }
      }
    }
  }
  n253 = control-ref of="总磷加标水杯定容体积"() -> (w69:refnum<vi>)
  n254 = control-ref of="氨氮加标水杯定容体积"() -> (w111:refnum<vi>)
  n255 = Unbundle By Name(w104) -> ("量程"=→"氨氮量程":dbl, "检出限"=→"氨氮检出限":dbl, "加标前水样浓度"=→"氨氮加标前水样浓度":dbl, "加标后水样浓度"=→"氨氮加标后水样浓度":dbl, "加标水杯定容体积"=→"氨氮加标水杯定容体积":dbl, "加标母液浓度"=→"氨氮母液浓度":dbl, "加标体积"=→"氨氮加标体积":dbl, "加标回收率"=→"氨氮加标回收率":dbl)
  n256 = control-ref of="总磷加标前水样浓度"() -> (w71:refnum<vi>)
  n257 = control-ref of="总磷加标后水样浓度"() -> (w70:refnum<vi>)
  n258 = control-ref of="氨氮加标前水样浓度"() -> (w112:refnum<vi>)
  n259 = control-ref of="氨氮加标后水样浓度"() -> (w108:refnum<vi>)
  n260 = control-ref of="COD加标回收率"() -> (w57:refnum<vi>)
  n261 = control-ref of="CODCr加标后水样浓度"() -> (w6:refnum<vi>)
  n262 = control-ref of="CODCr加标回收率"() -> (w2:refnum<vi>)
  n263 = control-ref of="CODCr加标前水样浓度"() -> (w7:refnum<vi>)
  n264 = control-ref of="CODCr加标水杯定容体积"() -> (w5:refnum<vi>)
  n265 = control-ref of="COD母液浓度"() -> (w59:refnum<vi>)
  n266 = control-ref of="COD加标体积"() -> (w58:refnum<vi>)
  n267 = control-ref of="CODCr检出限"() -> (w8:refnum<vi>)
  n268 = control-ref of="CODCr母液浓度"() -> (w4:refnum<vi>)
  n269 = control-ref of="CODCr量程"() -> (w9:refnum<vi>)
  n270 = control-ref of="CODCr加标体积"() -> (w3:refnum<vi>)
  n271 = call "质控参数读取.vi"("section"="总磷质控参数", "error in (no error)"=w85) -> ("error out"=w82:errorcluster, "参数"=w94:T8)  [unwired: 8 in]
  n272 = control-ref of="总磷加标回收率"() -> (w67:refnum<vi>)
  n273 = control-ref of="氨氮加标回收率"() -> (w106:refnum<vi>)
  n274 = control-ref of="COD检出限"() -> (w63:refnum<vi>)
  n275 = control-ref of="总磷母液浓度"() -> (w68:refnum<vi>)
  n276 = control-ref of="总磷加标体积"() -> (w66:refnum<vi>)
  n277 = control-ref of="氨氮母液浓度"() -> (w110:refnum<vi>)
  n278 = control-ref of="氨氮加标体积"() -> (w107:refnum<vi>)
  n279 = control-ref of="COD量程"() -> (w64:refnum<vi>)
  n280 = control-ref of="总磷检出限"() -> (w72:refnum<vi>)
  n281 = control-ref of="氨氮检出限"() -> (w113:refnum<vi>)
  n282 = control-ref of="总磷量程"() -> (w73:refnum<vi>)
  n283 = control-ref of="氨氮量程"() -> (w114:refnum<vi>)
  n284 = Build Array(w9, w8, w7, w6, w5, w4, w3, w2) -> (w1:refnum<vi>[])
  n285 = Obtain Notifier(name (unnamed)="采配水Process" ("名称（未命名）"), notification data type=FALSE) -> (notifier out=w48:refnum<notifier>)  [unwired: 2 in, 2 out]
  n286 = Build Array(w64, w63, w62, w61, w60, w59, w58, w57) -> (w56:refnum<vi>[])
  n287 = Build Array(w73, w72, w71, w70, w69, w68, w66, w67) -> (w65:refnum<vi>[])
  n288 = Build Array(w114, w113, w112, w108, w111, w110, w107, w106) -> (w109:refnum<vi>[])
  n289 = Unbundle By Name(w94) -> ("量程"=→"总磷量程":dbl, "检出限"=→"总磷检出限":dbl, "加标前水样浓度"=→"总磷加标前水样浓度":dbl, "加标后水样浓度"=→"总磷加标后水样浓度":dbl, "加标水杯定容体积"=→"总磷加标水杯定容体积":dbl, "加标母液浓度"=→"总磷母液浓度":dbl, "加标体积"=→"总磷加标体积":dbl, "加标回收率"=→"总磷加标回收率":dbl)
  n290 = call "质控参数读取.vi"("section"="COD质控参数", "error in (no error)"=w82) -> ("error out"=w33:errorcluster, "参数"=w84:T8)  [unwired: 8 in]
  n291 = Unbundle By Name(w84) -> ("量程"=→"COD量程":dbl, "检出限"=→"COD检出限":dbl, "加标前水样浓度"=→"COD加标前水样浓度":dbl, "加标后水样浓度"=→"COD加标后水样浓度":dbl, "加标水杯定容体积"=→"COD加标水杯定容体积":dbl, "加标母液浓度"=→"COD母液浓度":dbl, "加标体积"=→"COD加标体积":dbl, "加标回收率"=→"COD加标回收率":dbl)
  n292 = call "质控参数读取.vi"("section"="总氮质控参数", "error in (no error)"=w33) -> ("error out"=w18:errorcluster, "参数"=w32:T8)  [unwired: 8 in]
  n293 = Unbundle By Name(w32) -> ("量程"=→"总氮量程":dbl, "检出限"=→"总氮检出限":dbl, "加标前水样浓度"=→"总氮加标前水样浓度":dbl, "加标后水样浓度"=→"总氮加标后水样浓度":dbl, "加标水杯定容体积"=→"总氮加标水杯定容体积":dbl, "加标母液浓度"=→"总氮母液浓度":dbl, "加标体积"=→"总氮加标体积":dbl, "加标回收率"=→"总氮加标回收率":dbl)
  n294 = flat-sequence {
    frame #0 {
      w442 = "质控模块量程选择" ("section")
      w434 = "质控模块选择" ("section")
      w508 = "质控线性参数" ("section")
      w526 = "质控背隙补偿" ("section")
      n295 = call <vilib>:"Application Directory.vi"() -> ("Application Directory"=w532:path)
      n296 = Build Path(base path=w532, name or relative path="data\\Set.ini" ("名称或相对路径")) -> (appended path=w530:path)
      n297 = call <vilib>:"Open Config Data.vi"("configuration file path"=w530) -> ("error out"=w528:errorcluster, "refnum"=w529:T13)  [unwired: 8 in, 1 out]
      n298 = call-poly <vilib>:"Read Key.vi"("section"=w526, "error in (no error)"=w528, "key"="背隙值1", "refnum"=w529) -> ("error out"=w523:errorcluster, "value"=w518:i32, "refnum out"=w525:T13)  [unwired: 4 in, 1 out]
      n299 = local write "背隙补偿步数"(w518) -> ()
      n300 = call-poly <vilib>:"Read Key.vi"("section"=w526, "error in (no error)"=w523, "key"="背隙值2", "refnum"=w525) -> ("error out"=w521:errorcluster, "value"=w519:i32, "refnum out"=w522:T13)  [unwired: 4 in, 1 out]
      n301 = local write "背隙补偿步数 2"(w519) -> ()
      n302 = call-poly <vilib>:"Read Key.vi"("section"=w526, "error in (no error)"=w521, "key"="背隙值3", "refnum"=w522) -> ("error out"=w515:errorcluster, "value"=w517:i32, "refnum out"=w516:T13)  [unwired: 4 in, 1 out]
      n303 = local write "背隙补偿步数 3"(w517) -> ()
      n304 = call-poly <vilib>:"Read Key.vi"("section"=w508, "error in (no error)"=w515, "key"="标准体积1", "refnum"=w516) -> ("error out"=w511:errorcluster, "value"=w513:dbl, "refnum out"=w512:T13)  [unwired: 4 in, 1 out]
      n305 = local write "标准体积 1"(w513) -> ()
      n306 = call-poly <vilib>:"Read Key.vi"("section"=w508, "error in (no error)"=w511, "key"="标准体积2", "refnum"=w512) -> ("error out"=w509:errorcluster, "value"=w502:dbl, "refnum out"=w510:T13)  [unwired: 4 in, 1 out]
      n307 = local write "标准体积 2"(w502) -> ()
      n308 = call-poly <vilib>:"Read Key.vi"("section"=w508, "error in (no error)"=w509, "key"="标准体积3", "refnum"=w510) -> ("error out"=w506:errorcluster, "value"=w501:dbl, "refnum out"=w507:T13)  [unwired: 4 in, 1 out]
      n309 = local write "标准体积 3"(w501) -> ()
      n310 = call-poly <vilib>:"Read Key.vi"("section"=w508, "error in (no error)"=w506, "key"="标准体积4", "refnum"=w507) -> ("error out"=w504:errorcluster, "value"=w486:dbl, "refnum out"=w505:T13)  [unwired: 4 in, 1 out]
      n311 = local write "标准体积 4"(w486) -> ()
      n312 = Build Array("时间" ("table"), "参数" ("table"), "加标前水样测试时间" ("table"), "加标前水样浓度值" ("元素"), "加标后水样浓度值" ("元素"), "加标母液浓度值" ("元素"), "加标体积" ("元素"), "加标水杯定容体积" ("元素"), "加标回收率" ("元素")) -> (→"columns":string[])
      n313 = call-poly <vilib>:"Read Key.vi"("section"=w508, "error in (no error)"=w504, "key"="标准体积5", "refnum"=w505) -> ("error out"=w495:errorcluster, "value"=w485:dbl, "refnum out"=w496:T13)  [unwired: 4 in, 1 out]
      n314 = local write "标准体积 5"(w485) -> ()
      n315 = call-poly <vilib>:"Read Key.vi"("section"=w508, "error in (no error)"=w495, "key"="实际体积1", "refnum"=w496) -> ("error out"=w493:errorcluster, "value"=w484:dbl, "refnum out"=w494:T13)  [unwired: 4 in, 1 out]
      n316 = local write "实际体积 1"(w484) -> ()
      n317 = call-poly <vilib>:"Read Key.vi"("section"=w508, "error in (no error)"=w493, "key"="实际体积2", "refnum"=w494) -> ("error out"=w491:errorcluster, "value"=w483:dbl, "refnum out"=w492:T13)  [unwired: 4 in, 1 out]
      n318 = local write "实际体积 2"(w483) -> ()
      n319 = call-poly <vilib>:"Read Key.vi"("section"=w508, "error in (no error)"=w491, "key"="实际体积3", "refnum"=w492) -> ("error out"=w489:errorcluster, "value"=w480:dbl, "refnum out"=w490:T13)  [unwired: 4 in, 1 out]
      n320 = local write "实际体积 3"(w480) -> ()
      n321 = call-poly <vilib>:"Read Key.vi"("section"=w508, "error in (no error)"=w489, "key"="实际体积4", "refnum"=w490) -> ("error out"=w487:errorcluster, "value"=w479:dbl, "refnum out"=w488:T13)  [unwired: 4 in, 1 out]
      n322 = local write "实际体积 4"(w479) -> ()
      n323 = call-poly <vilib>:"Read Key.vi"("section"=w508, "error in (no error)"=w487, "key"="实际体积5", "refnum"=w488) -> ("error out"=w474:errorcluster, "value"=w478:dbl, "refnum out"=w475:T13)  [unwired: 4 in, 1 out]
      n324 = local write "实际体积 5"(w478) -> ()
      n325 = call-poly <vilib>:"Read Key.vi"("section"="质控手动体积选择", "error in (no error)"=w474, "key"="手动体积选择" ("section"), "refnum"=w475) -> ("error out"=w469:errorcluster, "value"=w471:i32, "refnum out"=w470:T13)  [unwired: 4 in, 1 out]
      n326 = local write "注出体积选择"(w471) -> ()
      n327 = call-poly <vilib>:"Read Key.vi"("section"=w434, "error in (no error)"=w469, "key"="模块1" ("section"), "refnum"=w470) -> ("error out"=w467:errorcluster, "value"=w459:bool, "refnum out"=w468:T13)  [unwired: 4 in, 1 out]
      n328 = local write "氨氮、总磷模块"(w459) -> ()
      n329 = call-poly <vilib>:"Read Key.vi"("section"=w434, "error in (no error)"=w467, "key"="模块2" ("section"), "refnum"=w468) -> ("error out"=w465:errorcluster, "value"=w460:bool, "refnum out"=w466:T13)  [unwired: 4 in, 1 out]
      n330 = local write "总氮模块选择"(w460) -> ()
      n331 = call-poly <vilib>:"Read Key.vi"("section"=w434, "error in (no error)"=w465, "key"="模块3" ("section"), "refnum"=w466) -> ("error out"=w436:errorcluster, "value"=w461:bool, "refnum out"=w437:T13)  [unwired: 4 in, 1 out]
      n332 = local write "CODMn选择"(w461) -> ()
      n333 = call-poly <vilib>:"Read Key.vi"("section"=w434, "error in (no error)"=w436, "key"="模块4", "refnum"=w437) -> ("error out"=w432:errorcluster, "value"=w431:bool, "refnum out"=w433:T13)  [unwired: 4 in, 1 out]
      n334 = local write "CODCr选择"(w431) -> ()
      n335 = call-poly <vilib>:"Read Key.vi"("section"=w442, "error in (no error)"=w432, "key"="氨氮" ("section"), "refnum"=w433) -> ("error out"=w457:errorcluster, "value"=w448:u32, "refnum out"=w458:T13)  [unwired: 4 in, 1 out]
      n336 = local write "氨氮量程选择"(w448) -> ()
      n337 = call-poly <vilib>:"Read Key.vi"("section"=w442, "error in (no error)"=w457, "key"="总氮" ("section"), "refnum"=w458) -> ("error out"=w455:errorcluster, "value"=w447:u32, "refnum out"=w456:T13)  [unwired: 4 in, 1 out]
      n338 = local write "总氮量程选择"(w447) -> ()
      n339 = call-poly <vilib>:"Read Key.vi"("section"=w442, "error in (no error)"=w455, "key"="总磷" ("section"), "refnum"=w456) -> ("error out"=w453:errorcluster, "value"=w446:u32, "refnum out"=w454:T13)  [unwired: 4 in, 1 out]
      n340 = local write "总磷量程选择"(w446) -> ()
      n341 = call-poly <vilib>:"Read Key.vi"("section"=w442, "error in (no error)"=w453, "key"="CODMn" ("section"), "refnum"=w454) -> ("error out"=w443:errorcluster, "value"=w445:u32, "refnum out"=w444:T13)  [unwired: 4 in, 1 out]
      n342 = local write "CODMn量程选择"(w445) -> ()
      n343 = call-poly <vilib>:"Read Key.vi"("section"=w442, "error in (no error)"=w443, "key"="CODCr" ("section"), "refnum"=w444) -> ("error out"=w439:errorcluster, "value"=w440:u32, "refnum out"=w438:T13)  [unwired: 4 in, 1 out]
      n344 = local write "CODCr量程选择"(w440) -> ()
      n345 = call <vilib>:"Close Config Data.vi"("error in (no error)"=w439, "refnum"=w438) -> ()  [unwired: 8 in, 2 out]
    }
  }
  n346 = Obtain Queue(name (unnamed)="采配水" ("名称（未命名）"), element data type=cluster{"命令":string, "数据":variant} {"命令"="", "数据"=variant}) -> (queue out=w45:refnum<queue>)  [unwired: 3 in, 2 out]
  n347 = while {
    tunnel: w109 -> [w549]
    tunnel: w65 -> [w548]
    tunnel: w56 -> [w547]
    tunnel: w48 -> [w546]
    tunnel: w45 -> [w545]
    tunnel: w35 -> [w544]
    tunnel: w1 -> [w543]
    stop <- FALSE stop-if-true
    # "氨氮站号是1，总磷总氮站号是2，COD站号是3"
    n348 = event shown="[37] \"加标回收\": 值改变" {
      selector: _ -> [_ _ _ _ _ _ _ _ _ _ _ _ _ _ _ _ _ _ _ _ _ _ _ _ _ _ _ _ _ _ _ _ _ _ _ _ _ _ _ _ _ _ _ _ _ _ _]
      dyn-events: _ -> [_ _ _ _ _ _ _ _ _ _ _ _ _ _ _ _ _ _ _ _ _ _ _ _ _ _ _ _ _ _ _ _ _ _ _ _ _ _ _ _ _ _ _ _ _ _ _]
      timeout: _ -> [_ _ _ _ _ _ _ _ _ _ _ _ _ _ _ _ _ _ _ _ _ _ _ _ _ _ _ _ _ _ _ _ _ _ _ _ _ _ _ _ _ _ _ _ _ _ _]
      tunnel: w549 -> [_ _ _ _ _ _ _ _ _ _ _ _ _ _ _ _ _ _ _ _ _ _ _ _ _ _ _ _ _ w912 _ _ _ _ w1009 _ _ _ _ _ _ _ _ _ _ _ _]
      tunnel: w548 -> [_ _ _ _ _ _ _ _ _ _ _ _ _ _ _ _ _ _ _ _ _ _ _ _ _ _ _ _ _ _ w926 _ _ _ w1006 _ _ _ _ _ _ _ _ _ _ _ _]
      tunnel: w547 -> [_ _ _ _ _ _ _ _ _ _ _ _ _ _ _ _ _ _ _ _ _ _ _ _ _ _ _ _ _ _ _ _ w964 w983 w1005 _ _ _ _ _ _ _ _ _ _ _ _]
      tunnel: w546 -> [_ _ _ _ _ _ _ _ _ _ _ _ _ _ _ _ _ _ _ _ _ _ _ _ _ _ _ _ _ _ _ _ _ _ _ _ _ w1038 _ _ _ _ _ w1199 w1230 _ _]
      tunnel: w545 -> [_ _ _ _ _ _ _ _ _ _ _ _ _ _ _ _ _ _ _ _ _ _ _ _ _ _ _ _ _ _ _ _ _ _ _ _ _ _ _ _ _ _ _ _ w1227 _ _]
      tunnel: w544 -> [_ _ _ _ _ _ _ _ _ _ _ _ _ _ _ _ _ _ _ _ _ _ _ _ _ _ _ _ _ _ _ w944 _ _ w1002 _ _ _ _ _ _ _ _ _ _ _ _]
      tunnel: [_ _ _ _ _ _ _ _ _ _ _ _ _ _ _ _ _ _ _ _ _ _ _ _ w837 w878 w885 w892 w899 _ _ _ _ _ _ _ _ _ w1068 _ _ _ _ _ _ _ _] -> _
      tunnel: w543 -> [_ _ _ _ _ _ _ _ _ _ _ _ _ _ _ _ _ _ _ _ _ _ _ _ _ _ _ _ _ _ _ _ _ _ w1001 _ _ _ _ _ _ _ _ _ _ _ _]
      event Timeout {
        n349 = event-data() -> ()  [unwired: 1 in, 3 out]
      }
      event "氨氮量程", "氨氮检出限", "氨氮加标前水样浓度", "氨氮加标水杯定容体积", "氨氮母液浓度", "氨氮加标后水样浓度": Mouse Down {
        n350 = event-data() -> ("CtlRef"=w554:refnum<vi>)  [unwired: 1 in, 7 out]
        n351 = property class="DigNum (严格)"(reference=w554) -> (reference out=w552:refnum<vi>, "Value"=w553:dbl)  [unwired: 1 in, 1 out]
        n352 = call "数字键盘.vi"("OldNumber"=w553) -> ("NewNumber"=w551:sgl)
        n353 = property class="DigNum (严格)"(reference=w552, "Val(Sgnl)"=w551) -> ()  [unwired: 1 in, 2 out]
      }
      event "总磷母液浓度", "总磷加标水杯定容体积", "总磷加标后水样浓度", "总磷加标前水样浓度", "总磷检出限", "总磷量程": Mouse Down {
        n354 = event-data() -> ("CtlRef"=w558:refnum<vi>)  [unwired: 1 in, 7 out]
        n355 = property class="DigNum (严格)"(reference=w558) -> (reference out=w556:refnum<vi>, "Value"=w557:dbl)  [unwired: 1 in, 1 out]
        n356 = call "数字键盘.vi"("OldNumber"=w557) -> ("NewNumber"=w555:sgl)
        n357 = property class="DigNum (严格)"(reference=w556, "Val(Sgnl)"=w555) -> ()  [unwired: 1 in, 2 out]
      }
      event "总氮母液浓度", "总氮加标水杯定容体积", "总氮加标后水样浓度", "总氮加标前水样浓度", "总氮检出限", "总氮量程": Mouse Down {
        n358 = event-data() -> ("CtlRef"=w562:refnum<vi>)  [unwired: 1 in, 7 out]
        n359 = property class="DigNum (严格)"(reference=w562) -> (reference out=w560:refnum<vi>, "Value"=w561:dbl)  [unwired: 1 in, 1 out]
        n360 = call "数字键盘.vi"("OldNumber"=w561) -> ("NewNumber"=w559:sgl)
        n361 = property class="DigNum (严格)"(reference=w560, "Val(Sgnl)"=w559) -> ()  [unwired: 1 in, 2 out]
      }
      event "COD母液浓度", "COD加标水杯定容体积", "COD加标后水样浓度", "COD加标前水样浓度", "COD检出限", "COD量程": Mouse Down {
        n362 = event-data() -> ("CtlRef"=w566:refnum<vi>)  [unwired: 1 in, 7 out]
        n363 = property class="DigNum (严格)"(reference=w566) -> (reference out=w564:refnum<vi>, "Value"=w565:dbl)  [unwired: 1 in, 1 out]
        n364 = call "数字键盘.vi"("OldNumber"=w565) -> ("NewNumber"=w563:sgl)
        n365 = property class="DigNum (严格)"(reference=w564, "Val(Sgnl)"=w563) -> ()  [unwired: 1 in, 2 out]
      }
      event "背隙补偿步数": Mouse Down {
        n366 = event-data() -> ()  [unwired: 1 in, 8 out]
        n367 = local read "背隙补偿步数"() -> (w568:i32)
        n368 = call "数字键盘.vi"("OldNumber"=w568) -> ("NewNumber"=w567:sgl)
        n369 = local write "背隙补偿步数"(w567) -> ()
      }
      event "标准体积 1": Mouse Down {
        n370 = event-data() -> ()  [unwired: 1 in, 8 out]
        n371 = local read "标准体积 1"() -> (w570:dbl)
        n372 = call "数字键盘.vi"("OldNumber"=w570) -> ("NewNumber"=w569:sgl)
        n373 = local write "标准体积 1"(w569) -> ()
      }
      event "标准体积 2": Mouse Down {
        n374 = event-data() -> ()  [unwired: 1 in, 8 out]
        n375 = local read "标准体积 2"() -> (w572:dbl)
        n376 = call "数字键盘.vi"("OldNumber"=w572) -> ("NewNumber"=w571:sgl)
        n377 = local write "标准体积 2"(w571) -> ()
      }
      event "标准体积 3": Mouse Down {
        n378 = event-data() -> ()  [unwired: 1 in, 8 out]
        n379 = local read "标准体积 3"() -> (w574:dbl)
        n380 = call "数字键盘.vi"("OldNumber"=w574) -> ("NewNumber"=w573:sgl)
        n381 = local write "标准体积 3"(w573) -> ()
      }
      event "标准体积 4": Mouse Down {
        n382 = event-data() -> ()  [unwired: 1 in, 8 out]
        n383 = local read "标准体积 4"() -> (w576:dbl)
        n384 = call "数字键盘.vi"("OldNumber"=w576) -> ("NewNumber"=w575:sgl)
        n385 = local write "标准体积 4"(w575) -> ()
      }
      event "标准体积 5": Mouse Down {
        n386 = event-data() -> ()  [unwired: 1 in, 8 out]
        n387 = local read "标准体积 5"() -> (w578:dbl)
        n388 = call "数字键盘.vi"("OldNumber"=w578) -> ("NewNumber"=w577:sgl)
        n389 = local write "标准体积 5"(w577) -> ()
      }
      event "实际体积 1": Mouse Down {
        n390 = event-data() -> ()  [unwired: 1 in, 8 out]
        n391 = local read "实际体积 1"() -> (w580:dbl)
        n392 = call "数字键盘.vi"("OldNumber"=w580) -> ("NewNumber"=w579:sgl)
        n393 = local write "实际体积 1"(w579) -> ()
      }
      event "实际体积 2": Mouse Down {
        n394 = event-data() -> ()  [unwired: 1 in, 8 out]
        n395 = local read "实际体积 2"() -> (w582:dbl)
        n396 = call "数字键盘.vi"("OldNumber"=w582) -> ("NewNumber"=w581:sgl)
        n397 = local write "实际体积 2"(w581) -> ()
      }
      event "实际体积 3": Mouse Down {
        n398 = event-data() -> ()  [unwired: 1 in, 8 out]
        n399 = local read "实际体积 3"() -> (w584:dbl)
        n400 = call "数字键盘.vi"("OldNumber"=w584) -> ("NewNumber"=w583:sgl)
        n401 = local write "实际体积 3"(w583) -> ()
      }
      event "实际体积 4": Mouse Down {
        n402 = event-data() -> ()  [unwired: 1 in, 8 out]
        n403 = local read "实际体积 4"() -> (w586:dbl)
        n404 = call "数字键盘.vi"("OldNumber"=w586) -> ("NewNumber"=w585:sgl)
        n405 = local write "实际体积 4"(w585) -> ()
      }
      event "实际体积 5": Mouse Down {
        n406 = event-data() -> ()  [unwired: 1 in, 8 out]
        n407 = local read "实际体积 5"() -> (w588:dbl)
        n408 = call "数字键盘.vi"("OldNumber"=w588) -> ("NewNumber"=w587:sgl)
        n409 = local write "实际体积 5"(w587) -> ()
      }
      event "K", "B", "K 2", "B 2", "K 3", "B 3", "K 4", "B 4": Mouse Down {
        n410 = event-data() -> ("CtlRef"=w592:refnum<vi>)  [unwired: 1 in, 7 out]
        n411 = property class="DigNum (严格)"(reference=w592) -> (reference out=w589:refnum<vi>, "Value"=w591:dbl)  [unwired: 1 in, 1 out]
        n412 = call "数字键盘.vi"("OldNumber"=w591) -> ("NewNumber"=w590:sgl)
        n413 = property class="DigNum (严格)"(reference=w589, "Value"=w590) -> ()  [unwired: 1 in, 2 out]
      }
      event "背隙补偿步数 2": Mouse Down {
        n414 = event-data() -> ()  [unwired: 1 in, 8 out]
        n415 = local read "背隙补偿步数 2"() -> (w593:i32)
        n416 = call "数字键盘.vi"("OldNumber"=w593) -> ("NewNumber"=w594:sgl)
        n417 = local write "背隙补偿步数 2"(w594) -> ()
      }
      event "背隙补偿步数 3": Mouse Down {
        n418 = event-data() -> ()  [unwired: 1 in, 8 out]
        n419 = local read "背隙补偿步数 3"() -> (w596:i32)
        n420 = call "数字键盘.vi"("OldNumber"=w596) -> ("NewNumber"=w595:sgl)
        n421 = local write "背隙补偿步数 3"(w595) -> ()
      }
      event "背隙补偿步数", "背隙补偿步数 2", "背隙补偿步数 3", "标准体积 1", "标准体积 2", "标准体积 3", "标准体积 4", "标准体积 5", "实际体积 1", "实际体积 2", "实际体积 3", "实际体积 4", "实际体积 5": Value Change {
        w617 = "质控线性参数" ("section")
        w648 = "质控背隙补偿" ("section")
        n422 = event-data() -> ()  [unwired: 1 in, 6 out]
        n423 = call <vilib>:"Application Directory.vi"() -> ("Application Directory"=w655:path)
        n424 = Build Path(base path=w655, name or relative path="data\\Set.ini" ("名称或相对路径")) -> (appended path=w653:path)
        n425 = call <vilib>:"Open Config Data.vi"("configuration file path"=w653) -> ("error out"=w651:errorcluster, "refnum"=w652:T13)  [unwired: 8 in, 1 out]
        n426 = call-poly <vilib>:"Write Key.vi"("section"=w648, "error in (no error)"=w651, "value"="背隙补偿步数", "key"="背隙值1", "refnum"=w652) -> ("error out"=w642:errorcluster, "refnum out"=w645:T13)  [unwired: 4 in, 1 out]
        n427 = call-poly <vilib>:"Write Key.vi"("section"=w648, "error in (no error)"=w642, "value"="背隙补偿步数 2", "key"="背隙值2", "refnum"=w645) -> ("error out"=w643:errorcluster, "refnum out"=w644:T13)  [unwired: 4 in, 1 out]
        n428 = local read "标准体积 1"() -> (w615:dbl)
        n429 = call-poly <vilib>:"Write Key.vi"("section"=w648, "error in (no error)"=w643, "value"="背隙补偿步数 3", "key"="背隙值3", "refnum"=w644) -> ("error out"=w638:errorcluster, "refnum out"=w639:T13)  [unwired: 4 in, 1 out]
        n430 = local read "标准体积 2"() -> (w614:dbl)
        n431 = local read "标准体积 3"() -> (w612:dbl)
        n432 = call-poly <vilib>:"Write Key.vi"("section"=w617, "error in (no error)"=w638, "value"=w615, "key"="标准体积1", "refnum"=w639) -> ("error out"=w636:errorcluster, "refnum out"=w637:T13)  [unwired: 4 in, 1 out]
        n433 = local read "标准体积 4"() -> (w608:dbl)
        n434 = call-poly <vilib>:"Write Key.vi"("section"=w617, "error in (no error)"=w636, "value"=w614, "key"="标准体积2", "refnum"=w637) -> ("error out"=w634:errorcluster, "refnum out"=w635:T13)  [unwired: 4 in, 1 out]
        n435 = call-poly <vilib>:"Write Key.vi"("section"=w617, "error in (no error)"=w634, "value"=w612, "key"="标准体积3", "refnum"=w635) -> ("error out"=w632:errorcluster, "refnum out"=w633:T13)  [unwired: 4 in, 1 out]
        n436 = local read "标准体积 5"() -> (w607:dbl)
        n437 = call-poly <vilib>:"Write Key.vi"("section"=w617, "error in (no error)"=w632, "value"=w608, "key"="标准体积4", "refnum"=w633) -> ("error out"=w630:errorcluster, "refnum out"=w631:T13)  [unwired: 4 in, 1 out]
        n438 = local read "实际体积 1"() -> (w601:dbl)
        n439 = call-poly <vilib>:"Write Key.vi"("section"=w617, "error in (no error)"=w630, "value"=w607, "key"="标准体积5", "refnum"=w631) -> ("error out"=w628:errorcluster, "refnum out"=w629:T13)  [unwired: 4 in, 1 out]
        n440 = local read "实际体积 2"() -> (w600:dbl)
        n441 = call-poly <vilib>:"Write Key.vi"("section"=w617, "error in (no error)"=w628, "value"=w601, "key"="实际体积1", "refnum"=w629) -> ("error out"=w626:errorcluster, "refnum out"=w627:T13)  [unwired: 4 in, 1 out]
        n442 = local read "实际体积 3"() -> (w599:dbl)
        n443 = local read "实际体积 4"() -> (w598:dbl)
        n444 = call-poly <vilib>:"Write Key.vi"("section"=w617, "error in (no error)"=w626, "value"=w600, "key"="实际体积2", "refnum"=w627) -> ("error out"=w624:errorcluster, "refnum out"=w625:T13)  [unwired: 4 in, 1 out]
        n445 = local read "实际体积 5"() -> (w597:dbl)
        n446 = call-poly <vilib>:"Write Key.vi"("section"=w617, "error in (no error)"=w624, "value"=w599, "key"="实际体积3", "refnum"=w625) -> ("error out"=w622:errorcluster, "refnum out"=w623:T13)  [unwired: 4 in, 1 out]
        n447 = call-poly <vilib>:"Write Key.vi"("section"=w617, "error in (no error)"=w622, "value"=w598, "key"="实际体积4", "refnum"=w623) -> ("error out"=w620:errorcluster, "refnum out"=w621:T13)  [unwired: 4 in, 1 out]
        n448 = call-poly <vilib>:"Write Key.vi"("section"=w617, "error in (no error)"=w620, "value"=w597, "key"="实际体积5", "refnum"=w621) -> ("error out"=w618:errorcluster, "refnum out"=w619:T13)  [unwired: 4 in, 1 out]
        n449 = call <vilib>:"Close Config Data.vi"("error in (no error)"=w618, "refnum"=w619) -> ()  [unwired: 8 in, 2 out]
      }
      event "氨氮、总磷模块", "总氮模块选择", "CODMn选择", "CODCr选择": Value Change {
        w659 = "质控模块选择" ("section")
        n450 = event-data() -> ()  [unwired: 1 in, 6 out]
        n451 = call <vilib>:"Application Directory.vi"() -> ("Application Directory"=w677:path)
        n452 = Build Path(base path=w677, name or relative path="data\\Set.ini" ("名称或相对路径")) -> (appended path=w675:path)
        n453 = local read "氨氮、总磷模块"() -> (w665:bool)
        n454 = call <vilib>:"Open Config Data.vi"("configuration file path"=w675) -> ("error out"=w673:errorcluster, "refnum"=w674:T13)  [unwired: 8 in, 1 out]
        n455 = local read "总氮模块选择"() -> (w664:bool)
        n456 = call-poly <vilib>:"Write Key.vi"("section"=w659, "error in (no error)"=w673, "value"=w665, "key"="模块1" ("section"), "refnum"=w674) -> ("error out"=w671:errorcluster, "refnum out"=w672:T13)  [unwired: 4 in, 1 out]
        n457 = local read "CODMn选择"() -> (w663:bool)
        n458 = call-poly <vilib>:"Write Key.vi"("section"=w659, "error in (no error)"=w671, "value"=w664, "key"="模块2" ("section"), "refnum"=w672) -> ("error out"=w669:errorcluster, "refnum out"=w670:T13)  [unwired: 4 in, 1 out]
        n459 = local read "CODCr选择"() -> (w656:bool)
        n460 = call-poly <vilib>:"Write Key.vi"("section"=w659, "error in (no error)"=w669, "value"=w663, "key"="模块3" ("section"), "refnum"=w670) -> ("error out"=w660:errorcluster, "refnum out"=w661:T13)  [unwired: 4 in, 1 out]
        n461 = call-poly <vilib>:"Write Key.vi"("section"=w659, "error in (no error)"=w660, "value"=w656, "key"="模块4" ("section"), "refnum"=w661) -> ("error out"=w657:errorcluster, "refnum out"=w658:T13)  [unwired: 4 in, 1 out]
        n462 = call <vilib>:"Close Config Data.vi"("error in (no error)"=w657, "refnum"=w658) -> ()  [unwired: 8 in, 2 out]
      }
      event "氨氮量程选择", "总氮量程选择", "总磷量程选择", "CODMn量程选择", "CODCr量程选择": Value Change {
        w684 = "质控模块量程选择" ("section")
        n463 = event-data() -> ()  [unwired: 1 in, 6 out]
        n464 = call <vilib>:"Application Directory.vi"() -> ("Application Directory"=w703:path)
        n465 = Build Path(base path=w703, name or relative path="data\\Set.ini" ("名称或相对路径")) -> (appended path=w701:path)
        n466 = local read "氨氮量程选择"() -> (w688:enum32{"H", "L", "AUTO"})
        n467 = call <vilib>:"Open Config Data.vi"("configuration file path"=w701) -> ("error out"=w699:errorcluster, "refnum"=w700:T13)  [unwired: 8 in, 1 out]
        n468 = local read "总氮量程选择"() -> (w687:enum32{"H", "L", "AUTO"})
        n469 = call-poly <vilib>:"Write Key.vi"("section"=w684, "error in (no error)"=w699, "value"=w688, "key"="氨氮" ("section"), "refnum"=w700) -> ("error out"=w697:errorcluster, "refnum out"=w698:T13)  [unwired: 4 in, 1 out]
        n470 = local read "总磷量程选择"() -> (w686:enum32{"H", "L", "AUTO"})
        n471 = call-poly <vilib>:"Write Key.vi"("section"=w684, "error in (no error)"=w697, "value"=w687, "key"="总氮" ("section"), "refnum"=w698) -> ("error out"=w695:errorcluster, "refnum out"=w696:T13)  [unwired: 4 in, 1 out]
        n472 = local read "CODMn量程选择"() -> (w685:enum32{"H", "L", "AUTO"})
        n473 = call-poly <vilib>:"Write Key.vi"("section"=w684, "error in (no error)"=w695, "value"=w686, "key"="总磷" ("section"), "refnum"=w696) -> ("error out"=w690:errorcluster, "refnum out"=w691:T13)  [unwired: 4 in, 1 out]
        n474 = call-poly <vilib>:"Write Key.vi"("section"=w684, "error in (no error)"=w690, "value"=w685, "key"="CODMn" ("section"), "refnum"=w691) -> ("error out"=w680:errorcluster, "refnum out"=w683:T13)  [unwired: 4 in, 1 out]
        n475 = local read "CODCr量程选择"() -> (w678:enum32{"H", "L", "AUTO"})
        n476 = call-poly <vilib>:"Write Key.vi"("section"=w684, "error in (no error)"=w680, "value"=w678, "key"="CODCr" ("section"), "refnum"=w683) -> ("error out"=w681:errorcluster, "refnum out"=w682:T13)  [unwired: 4 in, 1 out]
        n477 = call <vilib>:"Close Config Data.vi"("error in (no error)"=w681, "refnum"=w682) -> ()  [unwired: 8 in, 2 out]
      }
      event "写入": Value Change {
        n478 = event-data() -> ()  [unwired: 1 in, 6 out]
        n479 = local read "枚举"() -> (w705:enum16{"柱塞泵1", "柱塞泵2", "柱塞泵3", "柱塞泵4"})
        n480 = case shown="\"柱塞泵4\"" w705 {
          tunnel: [w706 w718 w729 w741] -> w704
          frame "柱塞泵1", Default {
            n481 = local read "K"() -> (w710:dbl)
            n482 = local read "B"() -> (w711:dbl)
            n483 = local read "背隙补偿步数"() -> (w707:i32)
            n484 = Build Array(w710, w711) -> (w712:dbl[])
            n485 = call "浮点转CDAB整形ZK.vi"("浮点数"=w712) -> ("CDAB整形输出"=w714:u16[])  [unwired: 10 in]
            n486 = Build Array(w707) -> (w713:i32[])
            n487 = Insert Into Array(array=w713, index=0 ("索引"), new element=w714) -> (w716:i32[])
            n488 = call "写入参数.vi"("values"=w716, "starting address"=u16 1, "Slave ID"=u8 1) -> ("error out"=w706:errorcluster)  [unwired: 8 in]
          }
          frame "柱塞泵2" {
            n489 = local read "背隙补偿步数 2"() -> (w720:i32)
            n490 = local read "K 2"() -> (w723:dbl)
            n491 = local read "B 2"() -> (w722:dbl)
            n492 = Build Array(w723, w722) -> (w724:dbl[])
            n493 = call "浮点转CDAB整形ZK.vi"("浮点数"=w724) -> ("CDAB整形输出"=w725:u16[])  [unwired: 10 in]
            n494 = Build Array(w720) -> (w719:i32[])
            n495 = Insert Into Array(array=w719, index=0 ("索引"), new element=w725) -> (w727:i32[])
            n496 = call "写入参数.vi"("values"=w727, "starting address"=u16 1, "Slave ID"=u8 2) -> ("error out"=w718:errorcluster)  [unwired: 8 in]
          }
          frame "柱塞泵3" {
            n497 = local read "背隙补偿步数 3"() -> (w731:i32)
            n498 = local read "K 3"() -> (w735:dbl)
            n499 = local read "B 3"() -> (w736:dbl)
            n500 = Build Array(w735, w736) -> (w737:dbl[])
            n501 = call "浮点转CDAB整形ZK.vi"("浮点数"=w737) -> ("CDAB整形输出"=w738:u16[])  [unwired: 10 in]
            n502 = Build Array(w731) -> (w733:i32[])
            n503 = Insert Into Array(array=w733, index=0 ("索引"), new element=w738) -> (w732:i32[])
            n504 = call "写入参数.vi"("values"=w732, "starting address"=u16 1, "Slave ID"=u8 3) -> ("error out"=w729:errorcluster)  [unwired: 8 in]
          }
          frame "柱塞泵4" {
            n505 = local read "K 4"() -> (w746:dbl)
            n506 = local read "B 4"() -> (w747:dbl)
            n507 = Build Array(w746, w747) -> (w748:dbl[])
            n508 = call "浮点转CDAB整形ZK.vi"("浮点数"=w748) -> ("CDAB整形输出"=w749:u16[])  [unwired: 10 in]
            n509 = Build Array(0 ("背隙补偿步数")) -> (w744:i32[])
            n510 = Insert Into Array(array=w744, index=0 ("索引"), new element=w749) -> (w743:i32[])
            n511 = call "写入参数.vi"("values"=w743, "starting address"=u16 1, "Slave ID"=u8 4) -> ("error out"=w741:errorcluster)  [unwired: 8 in]
          }
        }
        n512 = case shown="无错误" w704 {
          frame No Error {
            n513 = One Button Dialog(message="写入成功" ("消息"), button name ("OK")="确定" ("按钮名称（“确定”）")) -> ()  [unwired: 1 out]
          }
          frame Error {
            n514 = One Button Dialog(message="写入失败" ("消息"), button name ("OK")="确定" ("按钮名称（“确定”）")) -> ()  [unwired: 1 out]
          }
        }
      }
      event "读取": Value Change {
        n515 = event-data() -> ()  [unwired: 1 in, 6 out]
        n516 = local read "氨氮、总磷模块"() -> (w761:bool)
        n517 = case shown="假" w761 {
          tunnel: [errorcluster {"status"=FALSE, "code"=0, "source"=""} ("error out") w793] -> w771
          tunnel: [w786 w790] -> w769
          tunnel: [w785 w789] -> w768
          frame False {
            n518 = local read "线性值"() -> (w787:T1)
            n519 = Unbundle By Name(w787) -> ("K3"=w786:sgl, "B3"=w785:sgl)
          }
          frame True {
            n520 = call "读取参数.vi"("Slave ID"=u8 1, "starting address"=u16 1, "quantity"=u16 4) -> ("values"=w792:u16[], "error out"=w793:errorcluster)  [unwired: 6 in]
            n521 = call "浮点CDAB转换质控.vi"("数组"=w792) -> ("数组 2"=w791:sgl[])  [unwired: 10 in]
            n522 = Index Array(array=w791) -> (element #1=w790:sgl, element #2=w789:sgl)  [unwired: 2 in]
          }
        }
        n523 = local read "总氮模块选择"() -> (w762:bool)
        n524 = case shown="假" w762 {
          tunnel: w771 -> [w797 w808]
          tunnel: [w797 w807] -> w770
          tunnel: [w799 w804] -> w767
          tunnel: [w798 w803] -> w766
          frame False {
            n525 = local read "线性值"() -> (w800:T1)
            n526 = Unbundle By Name(w800) -> ("K3"=w799:sgl, "B3"=w798:sgl)
          }
          frame True {
            n527 = call "读取参数.vi"("Slave ID"=u8 2, "starting address"=u16 1, "quantity"=u16 4, "Error in"=w808) -> ("values"=w806:u16[], "error out"=w807:errorcluster)  [unwired: 5 in]
            n528 = call "浮点CDAB转换质控.vi"("数组"=w806) -> ("数组 2"=w805:sgl[])  [unwired: 10 in]
            n529 = Index Array(array=w805) -> (element #1=w804:sgl, element #2=w803:sgl)  [unwired: 2 in]
          }
        }
        n530 = local read "CODMn选择"() -> (w763:bool)
        n531 = case shown="假" w763 {
          tunnel: w770 -> [w810 w821]
          tunnel: [w812 w818] -> w765
          tunnel: [w811 w817] -> w764
          tunnel: [w810 w814] -> w759
          frame False {
            n532 = local read "线性值"() -> (w813:T1)
            n533 = Unbundle By Name(w813) -> ("K3"=w812:sgl, "B3"=w811:sgl)
          }
          frame True {
            n534 = call "读取参数.vi"("Slave ID"=u8 3, "starting address"=u16 1, "quantity"=u16 4, "Error in"=w821) -> ("values"=w820:u16[], "error out"=w814:errorcluster)  [unwired: 5 in]
            n535 = call "浮点CDAB转换质控.vi"("数组"=w820) -> ("数组 2"=w819:sgl[])  [unwired: 10 in]
            n536 = Index Array(array=w819) -> (element #1=w818:sgl, element #2=w817:sgl)  [unwired: 2 in]
          }
        }
        n537 = local read "CODCr选择"() -> (w757:bool)
        n538 = case shown="真" w757 {
          tunnel: w759 -> [w772 w783]
          tunnel: [w774 w780] -> w756
          tunnel: [w773 w779] -> w755
          tunnel: [w772 w776] -> w758
          frame False {
            n539 = local read "线性值"() -> (w775:T1)
            n540 = Unbundle By Name(w775) -> ("K4"=w774:sgl, "B4"=w773:sgl)
          }
          frame True {
            n541 = call "读取参数.vi"("Slave ID"=u8 4, "starting address"=u16 1, "quantity"=u16 4, "Error in"=w783) -> ("values"=w782:u16[], "error out"=w776:errorcluster)  [unwired: 5 in]
            n542 = call "浮点CDAB转换质控.vi"("数组"=w782) -> ("数组 2"=w781:sgl[])  [unwired: 10 in]
            n543 = Index Array(array=w781) -> (element #1=w780:sgl, element #2=w779:sgl)  [unwired: 2 in]
          }
        }
        n544 = Bundle By Name(cluster=T1 {"K1"=0.0, "B1"=0.0, "K2"=0.0, "B2"=0.0, "K3"=0.0, "B3"=0.0, "K4"=0.0, "B4"=0.0} ("线性值"), "K1"=w769, "B1"=w768, "K2"=w767, "B2"=w766, "K3"=w765, "B3"=w764, "K4"=w756, "B4"=w755) -> (→"线性值":T1)
        n545 = case shown="无错误" w758 {
          frame No Error {
            n546 = One Button Dialog(message="读取成功" ("消息"), button name ("OK")="确定" ("按钮名称（“确定”）")) -> ()  [unwired: 1 out]
          }
          frame Error {
            n547 = One Button Dialog(message="读取失败" ("消息"), button name ("OK")="确定" ("按钮名称（“确定”）")) -> ()  [unwired: 1 out]
          }
        }
      }
      event "注出体积选择": Value Change {
        n548 = event-data() -> ()  [unwired: 1 in, 6 out]
        n549 = case shown="0" "注出体积选择" {
          tunnel: [0.1 0.3 0.5 0.8 1.0] -> w847
          frame 0 {
          }
          frame 1 {
          }
          frame 2 {
          }
          frame 3 {
          }
          frame 4, Default {
          }
        }
        n550 = local read "氨氮、总磷模块"() -> (w834:bool)
        n551 = Build Array(w847) -> (w835:dbl[])
        n552 = call "浮点转CDAB整形ZK.vi"("浮点数"=w835) -> ("CDAB整形输出"=w828:u16[])  [unwired: 10 in]
        n553 = case shown="真" w834 {
          tunnel: [_ w859] -> w849
          tunnel: [u16 8 ("starting address") w858] -> w830
          tunnel: w828 -> [_ w857]
          frame False {
          }
          frame True {
            w858 = u16 8 ("starting address")
            n554 = call "写入参数.vi"("values"=w857, "starting address"=w858, "Slave ID"=u8 1) -> ("error out"=w859:errorcluster)  [unwired: 8 in]
          }
        }
        n555 = local read "总氮模块选择"() -> (w833:bool)
        n556 = case shown="真" w833 {
          tunnel: w849 -> [w861 w865]
          tunnel: [w861 w864] -> w848
          tunnel: w830 -> [_ w863]
          tunnel: w828 -> [_ w862]
          frame False {
          }
          frame True {
            n557 = call "写入参数.vi"("Error in"=w865, "values"=w862, "starting address"=w863, "Slave ID"=u8 2) -> ("error out"=w864:errorcluster)  [unwired: 7 in]
          }
        }
        n558 = local read "CODMn选择"() -> (w832:bool)
        n559 = case shown="真" w832 {
          tunnel: w848 -> [w867 w871]
          tunnel: w830 -> [_ w870]
          tunnel: [w867 w869] -> w829
          tunnel: w828 -> [_ w868]
          frame False {
          }
          frame True {
            n560 = call "写入参数.vi"("Error in"=w871, "values"=w868, "starting address"=w870, "Slave ID"=u8 3) -> ("error out"=w869:errorcluster)  [unwired: 7 in]
          }
        }
        n561 = local read "CODCr选择"() -> (w831:bool)
        n562 = case shown="真" w831 {
          tunnel: w829 -> [w850 w854]
          tunnel: w830 -> [_ w853]
          tunnel: [w850 w852] -> w827
          tunnel: w828 -> [_ w851]
          frame False {
          }
          frame True {
            n563 = call "写入参数.vi"("Error in"=w854, "values"=w851, "starting address"=w853, "Slave ID"=u8 4) -> ("error out"=w852:errorcluster)  [unwired: 7 in]
          }
        }
        n564 = call <vilib>:"Application Directory.vi"() -> ("Application Directory"=w846:path)
        n565 = Build Path(base path=w846, name or relative path="data\\Set.ini" ("名称或相对路径")) -> (appended path=w844:path)
        n566 = call <vilib>:"Open Config Data.vi"("error in (no error)"=w827, "configuration file path"=w844) -> ("error out"=w840:errorcluster, "refnum"=w841:T13)  [unwired: 7 in, 1 out]
        n567 = call-poly <vilib>:"Write Key.vi"("section"="质控手动体积选择", "error in (no error)"=w840, "value"="注出体积选择", "key"="手动体积选择" ("section"), "refnum"=w841) -> ("error out"=w842:errorcluster, "refnum out"=w843:T13)  [unwired: 4 in, 1 out]
        n568 = call <vilib>:"Close Config Data.vi"("error in (no error)"=w842, "refnum"=w843) -> ("error out"=w837:errorcluster)  [unwired: 8 in, 1 out]
      }
      event "柱塞泵1": Value Change {
        n569 = event-data() -> ()  [unwired: 1 in, 6 out]
        n570 = Build Array("柱塞泵1") -> (w879:bool[])
        n571 = call "多个线圈写入.vi"("values"=w879, "starting address"=u16 2104, "Slave ID"=u8 1) -> ("error out"=w878:errorcluster)  [unwired: 8 in]
        n572 = case shown="错误" w878 {
          frame No Error {
          }
          frame Error {
            n573 = One Button Dialog(message="启动失败" ("消息"), button name ("OK")="确定" ("按钮名称（“确定”）")) -> ()  [unwired: 1 out]
          }
        }
      }
      event "柱塞泵2": Value Change {
        n574 = event-data() -> ()  [unwired: 1 in, 6 out]
        n575 = Build Array("柱塞泵2") -> (w887:bool[])
        n576 = call "多个线圈写入.vi"("values"=w887, "starting address"=u16 2104, "Slave ID"=u8 2) -> ("error out"=w885:errorcluster)  [unwired: 8 in]
        n577 = case shown="错误" w885 {
          frame No Error {
          }
          frame Error {
            n578 = One Button Dialog(message="启动失败" ("消息"), button name ("OK")="确定" ("按钮名称（“确定”）")) -> ()  [unwired: 1 out]
          }
        }
      }
      event "柱塞泵3": Value Change {
        n579 = event-data() -> ()  [unwired: 1 in, 6 out]
        n580 = Build Array("柱塞泵3") -> (w894:bool[])
        n581 = call "多个线圈写入.vi"("values"=w894, "starting address"=u16 2104, "Slave ID"=u8 3) -> ("error out"=w892:errorcluster)  [unwired: 8 in]
        n582 = case shown="无错误" w892 {
          frame No Error {
          }
          frame Error {
            n583 = One Button Dialog(message="启动失败" ("消息"), button name ("OK")="确定" ("按钮名称（“确定”）")) -> ()  [unwired: 1 out]
          }
        }
      }
      event "柱塞泵4": Value Change {
        n584 = event-data() -> ()  [unwired: 1 in, 6 out]
        n585 = Build Array("柱塞泵4") -> (w901:bool[])
        n586 = call "多个线圈写入.vi"("values"=w901, "starting address"=u16 2104, "Slave ID"=u8 4) -> ("error out"=w899:errorcluster)  [unwired: 8 in]
        n587 = case shown="无错误" w899 {
          frame No Error {
          }
          frame Error {
            n588 = One Button Dialog(message="启动失败" ("消息"), button name ("OK")="确定" ("按钮名称（“确定”）")) -> ()  [unwired: 1 out]
          }
        }
      }
      event "氨氮量程", "氨氮检出限", "氨氮加标前水样浓度", "氨氮母液浓度", "氨氮加标水杯定容体积", "氨氮加标后水样浓度": Value Change {
        n589 = event-data() -> ()  [unwired: 1 in, 6 out]
        n590 = for {
          tunnel: w912 -> [w924] mode=indexing
          tunnel: [w923] -> w921 mode=indexing
          n591 = property class="DigNum (严格)"(reference=w924) -> ("Value"=w923:dbl)  [unwired: 1 in, 2 out]
        }
        n592 = Index Array(array=w921) -> (element #1=w920:dbl, element #2=w919:dbl, element #3=w906:dbl, element #4=w918:dbl, element #5=w917:dbl, element #6=w915:dbl)  [unwired: 6 in]
        n593 = Bundle By Name(cluster=T8 {"量程"=0.0, "检出限"=0.0, "加标前水样浓度"=0.0, "加标后水样浓度"=0.0, "加标水杯定容体积"=0.0, "加标母液浓度"=0.0, "加标体积"=0.0, "加标回收率"=0.0} ("参数"), "量程"=w920, "检出限"=w919, "加标前水样浓度"=w906, "加标后水样浓度"=w918, "加标水杯定容体积"=w917, "加标母液浓度"=w915) -> (w914:T8)
        n594 = global write "水样浓度全局.vi" "氨氮加标前水样浓度"(w906) -> ()
        n595 = call "加标回收率计算.vi"("参数"=w914) -> ("参数 out"=w913:T8)  [unwired: 10 in]
        n596 = Index Array(array=w912, index #1=6 ("索引")) -> (element #1=w911:refnum<vi>, element #2=w909:refnum<vi>)  [unwired: 1 in]
        n597 = call "质控参数保存.vi"("section"="氨氮质控参数", "参数"=w913) -> ()  [unwired: 9 in, 1 out]
        n598 = Unbundle By Name(w913) -> ("加标体积"=w907:dbl, "加标回收率"=w908:dbl)
        n599 = property class="DigNum (严格)"(reference=w911, "Value"=w907) -> ()  [unwired: 1 in, 2 out]
        n600 = property class="DigNum (严格)"(reference=w909, "Value"=w908) -> ()  [unwired: 1 in, 2 out]
      }
      event "总磷母液浓度", "总磷加标水杯定容体积", "总磷加标后水样浓度", "总磷加标前水样浓度", "总磷检出限", "总磷量程": Value Change {
        n601 = event-data() -> ()  [unwired: 1 in, 6 out]
        n602 = for {
          tunnel: w926 -> [w943] mode=indexing
          tunnel: [w942] -> w940 mode=indexing
          n603 = property class="DigNum (严格)"(reference=w943) -> ("Value"=w942:dbl)  [unwired: 1 in, 2 out]
        }
        n604 = Index Array(array=w940) -> (element #1=w939:dbl, element #2=w938:dbl, element #3=w925:dbl, element #4=w937:dbl, element #5=w936:dbl, element #6=w934:dbl)  [unwired: 6 in]
        n605 = global write "水样浓度全局.vi" "总磷加标前水样浓度"(w925) -> ()
        n606 = Bundle By Name(cluster=T8 {"量程"=0.0, "检出限"=0.0, "加标前水样浓度"=0.0, "加标后水样浓度"=0.0, "加标水杯定容体积"=0.0, "加标母液浓度"=0.0, "加标体积"=0.0, "加标回收率"=0.0} ("参数"), "量程"=w939, "检出限"=w938, "加标前水样浓度"=w925, "加标后水样浓度"=w937, "加标水杯定容体积"=w936, "加标母液浓度"=w934) -> (w933:T8)
        n607 = call "加标回收率计算.vi"("参数"=w933) -> ("参数 out"=w932:T8)  [unwired: 10 in]
        n608 = Index Array(array=w926, index #1=6 ("索引")) -> (element #1=w931:refnum<vi>, element #2=w928:refnum<vi>)  [unwired: 1 in]
        n609 = call "质控参数保存.vi"("section"="总磷质控参数", "参数"=w932) -> ()  [unwired: 9 in, 1 out]
        n610 = Unbundle By Name(w932) -> ("加标体积"=w929:dbl, "加标回收率"=w927:dbl)
        n611 = property class="DigNum (严格)"(reference=w931, "Value"=w929) -> ()  [unwired: 1 in, 2 out]
        n612 = property class="DigNum (严格)"(reference=w928, "Value"=w927) -> ()  [unwired: 1 in, 2 out]
      }
      event "总氮量程", "总氮检出限", "总氮加标前水样浓度", "总氮加标后水样浓度", "总氮加标水杯定容体积", "总氮母液浓度": Value Change {
        n613 = event-data() -> ()  [unwired: 1 in, 6 out]
        n614 = for {
          tunnel: w944 -> [w962] mode=indexing
          tunnel: [w961] -> w959 mode=indexing
          n615 = property class="DigNum (严格)"(reference=w962) -> ("Value"=w961:dbl)  [unwired: 1 in, 2 out]
        }
        n616 = Index Array(array=w959) -> (element #1=w958:dbl, element #2=w957:dbl, element #3=w945:dbl, element #4=w956:dbl, element #5=w955:dbl, element #6=w953:dbl)  [unwired: 6 in]
        n617 = global write "水样浓度全局.vi" "总氮加标前水样浓度"(w945) -> ()
        n618 = Bundle By Name(cluster=T8 {"量程"=0.0, "检出限"=0.0, "加标前水样浓度"=0.0, "加标后水样浓度"=0.0, "加标水杯定容体积"=0.0, "加标母液浓度"=0.0, "加标体积"=0.0, "加标回收率"=0.0} ("参数"), "量程"=w958, "检出限"=w957, "加标前水样浓度"=w945, "加标后水样浓度"=w956, "加标水杯定容体积"=w955, "加标母液浓度"=w953) -> (w952:T8)
        n619 = call "加标回收率计算.vi"("参数"=w952) -> ("参数 out"=w951:T8)  [unwired: 10 in]
        n620 = Index Array(array=w944, index #1=6 ("索引")) -> (element #1=w950:refnum<vi>, element #2=w947:refnum<vi>)  [unwired: 1 in]
        n621 = call "质控参数保存.vi"("section"="总氮质控参数", "参数"=w951) -> ()  [unwired: 9 in, 1 out]
        n622 = Unbundle By Name(w951) -> ("加标体积"=w948:dbl, "加标回收率"=w946:dbl)
        n623 = property class="DigNum (严格)"(reference=w950, "Value"=w948) -> ()  [unwired: 1 in, 2 out]
        n624 = property class="DigNum (严格)"(reference=w947, "Value"=w946) -> ()  [unwired: 1 in, 2 out]
      }
      event "COD母液浓度", "COD加标水杯定容体积", "COD加标后水样浓度", "COD加标前水样浓度", "COD检出限", "COD量程": Value Change {
        n625 = event-data() -> ()  [unwired: 1 in, 6 out]
        n626 = for {
          tunnel: w964 -> [w981] mode=indexing
          tunnel: [w980] -> w978 mode=indexing
          n627 = property class="DigNum (严格)"(reference=w981) -> ("Value"=w980:dbl)  [unwired: 1 in, 2 out]
        }
        n628 = Index Array(array=w978) -> (element #1=w977:dbl, element #2=w976:dbl, element #3=w963:dbl, element #4=w975:dbl, element #5=w974:dbl, element #6=w972:dbl)  [unwired: 6 in]
        n629 = global write "水样浓度全局.vi" "COD加标前水样浓度"(w963) -> ()
        n630 = Bundle By Name(cluster=T8 {"量程"=0.0, "检出限"=0.0, "加标前水样浓度"=0.0, "加标后水样浓度"=0.0, "加标水杯定容体积"=0.0, "加标母液浓度"=0.0, "加标体积"=0.0, "加标回收率"=0.0} ("参数"), "量程"=w977, "检出限"=w976, "加标前水样浓度"=w963, "加标后水样浓度"=w975, "加标水杯定容体积"=w974, "加标母液浓度"=w972) -> (w971:T8)
        n631 = call "加标回收率计算.vi"("参数"=w971) -> ("参数 out"=w970:T8)  [unwired: 10 in]
        n632 = Index Array(array=w964, index #1=6 ("索引")) -> (element #1=w969:refnum<vi>, element #2=w966:refnum<vi>)  [unwired: 1 in]
        n633 = call "质控参数保存.vi"("section"="COD质控参数", "参数"=w970) -> ()  [unwired: 9 in, 1 out]
        n634 = Unbundle By Name(w970) -> ("加标体积"=w967:dbl, "加标回收率"=w965:dbl)
        n635 = property class="DigNum (严格)"(reference=w969, "Value"=w967) -> ()  [unwired: 1 in, 2 out]
        n636 = property class="DigNum (严格)"(reference=w966, "Value"=w965) -> ()  [unwired: 1 in, 2 out]
      }
      event "CODCr母液浓度", "CODCr加标水杯定容体积", "CODCr加标前水样浓度", "CODCr检出限", "CODCr量程", "CODCr加标后水样浓度": Value Change {
        n637 = event-data() -> ()  [unwired: 1 in, 6 out]
        n638 = for {
          tunnel: w983 -> [w1000] mode=indexing
          tunnel: [w999] -> w997 mode=indexing
          n639 = property class="DigNum (严格)"(reference=w1000) -> ("Value"=w999:dbl)  [unwired: 1 in, 2 out]
        }
        n640 = Index Array(array=w997) -> (element #1=w996:dbl, element #2=w995:dbl, element #3=w982:dbl, element #4=w994:dbl, element #5=w993:dbl, element #6=w991:dbl)  [unwired: 6 in]
        n641 = global write "水样浓度全局.vi" "CODCr加标前水样浓度"(w982) -> ()
        n642 = Bundle By Name(cluster=T8 {"量程"=0.0, "检出限"=0.0, "加标前水样浓度"=0.0, "加标后水样浓度"=0.0, "加标水杯定容体积"=0.0, "加标母液浓度"=0.0, "加标体积"=0.0, "加标回收率"=0.0} ("参数"), "量程"=w996, "检出限"=w995, "加标前水样浓度"=w982, "加标后水样浓度"=w994, "加标水杯定容体积"=w993, "加标母液浓度"=w991) -> (w990:T8)
        n643 = call "加标回收率计算.vi"("参数"=w990) -> ("参数 out"=w989:T8)  [unwired: 10 in]
        n644 = Index Array(array=w983, index #1=6 ("索引")) -> (element #1=w988:refnum<vi>, element #2=w985:refnum<vi>)  [unwired: 1 in]
        n645 = call "质控参数保存.vi"("section"="CODCr质控参数", "参数"=w989) -> ()  [unwired: 9 in, 1 out]
        n646 = Unbundle By Name(w989) -> ("加标体积"=w986:dbl, "加标回收率"=w984:dbl)
        n647 = property class="DigNum (严格)"(reference=w988, "Value"=w986) -> ()  [unwired: 1 in, 2 out]
        n648 = property class="DigNum (严格)"(reference=w985, "Value"=w984) -> ()  [unwired: 1 in, 2 out]
      }
      event "氨氮调试", "总磷调试", "CODMn调试", "总氮调试", "CODCr调试": Value Change {
        n649 = event-data() -> ("CtlRef"=w1008:refnum<vi>)  [unwired: 1 in, 5 out]
        n650 = property class="Bool"(reference=w1008) -> ("Label.Text"=w1007:string)  [unwired: 1 in, 2 out]
        n651 = case shown="\"CODCr调试\"" w1007 {
          tunnel: w1009 -> [w1010 _ _ _ _]
          tunnel: w1006 -> [_ w1012 _ _ _]
          tunnel: w1005 -> [_ _ _ w1016 _]
          tunnel: ["氨氮模块" ("标题") "总磷模块" ("标题") "总氮模块" ("标题") "CODMn模块" ("标题") "CODCr模块" ("标题")] -> w1004
          tunnel: [w1010 w1012 w1014 w1016 w1018] -> w1003
          tunnel: w1002 -> [_ _ w1014 _ _]
          tunnel: w1001 -> [_ _ _ _ w1018]
          frame "氨氮调试", Default {
          }
          frame "总磷调试" {
          }
          frame "总氮调试" {
          }
          frame "CODMn调试" {
          }
          frame "CODCr调试" {
          }
        }
        n652 = call "加标模块单控对话框.vi"("数组"=w1003, "标题"=w1004) -> ()  [unwired: 10 in]
      }
      event "氨氮停止", "总磷停止", "CODMn停止", "总氮停止", "CODCr停止": Value Change {
        n653 = event-data() -> ("CtlRef"=w1024:refnum<vi>)  [unwired: 1 in, 5 out]
        n654 = property class="Bool"(reference=w1024) -> ("Label.Text"=w1023:string)  [unwired: 1 in, 2 out]
        n655 = case shown="\"CODCr模块\"" w1023 {
          tunnel: [u8 1 ("Slave ID") u8 2 ("Slave ID") u8 3 ("Slave ID") u8 4 ("Slave ID")] -> w1020
          frame "氨氮停止", Default {
          }
          frame "总氮停止", "总磷停止" {
          }
          frame "CODMn停止" {
          }
          frame "CODCr模块" {
          }
        }
        n656 = call "单个写入.vi"("value"=u16 2, "address"=u16 103, "Slave ID"=w1020) -> ()  [unwired: 8 in, 1 out]
      }
      event "氨氮排液", "CODMn排液", "总磷排液", "总氮排液", "CODCr排液": Value Change {
        n657 = event-data() -> ("CtlRef"=w1033:refnum<vi>)  [unwired: 1 in, 5 out]
        n658 = property class="Bool"(reference=w1033) -> ("Label.Text"=w1032:string)  [unwired: 1 in, 2 out]
        n659 = case shown="\"CODCr模块\"" w1032 {
          tunnel: [u8 1 ("Slave ID") u8 2 ("Slave ID") u8 3 ("Slave ID") u8 4 ("Slave ID")] -> w1029
          frame "氨氮排液", Default {
          }
          frame "总氮排液", "总磷排液" {
          }
          frame "CODMn排液" {
          }
          frame "CODCr模块" {
          }
        }
        n660 = call "单个写入.vi"("value"=u16 3, "address"=u16 103, "Slave ID"=w1029) -> ()  [unwired: 8 in, 1 out]
      }
      event "加标回收": Value Change {
        n661 = event-data() -> ()  [unwired: 1 in, 6 out]
        n662 = flat-sequence {
          tunnel: [w1042] -> w1041
          tunnel: [w1046] -> w1040
          tunnel: [w1045] -> w1039
          tunnel: w1038 -> [w1043]
          tunnel: w1041 -> [w1054]
          tunnel: w1040 -> [w1053]
          tunnel: w1039 -> [w1052]
          frame #0 {
            n663 = Send Notification(notification=FALSE ("通知"), notifier=w1043) -> ()  [unwired: 1 in, 2 out]
            n664 = call "质控启动流程对话框.vi"() -> ("启动模块"=w1042:T3, "直接启动"=w1045:bool, "常规启动"=w1046:bool)  [unwired: 8 in, 1 out]
            "常规启动" <- w1046
            "直接启动" <- w1045
            "启动模块" <- w1042
          }
          frame #1 {
            n665 = Bundle By Name(cluster=T6 {"是否启用仪器"=FALSE, "CODMn"={"启动测量模式"={"测量模式"=enum."水样测量"}, "确定按钮"=FALSE}, "启动模块 3"={"氨氮"=FALSE, "总磷"=FALSE, "总氮"=FALSE, "COD"=FALSE}, "常规启动"=FALSE, "直接启动"=FALSE} ("输出簇"), "是否启用仪器"=TRUE, "启动模块 3"=w1054, "常规启动"=w1053, "直接启动"=w1052) -> (w1047:T6)
            "输出簇" <- w1047
            n666 = vi-ref "质控单元.lvlib:一体站流程质控自动启动.vi"() -> (w1050:refnum<vi>)
            n667 = property class="VI"(reference=w1050) -> ("Name"=w1051:string, "Exec.State"=w1049:T16)  [unwired: 1 in, 2 out]
            n668 = case shown="\"Idle\"" w1049 {
              tunnel: w1051 -> [_ w1066]
              tunnel: w1047 -> [_ w1065]
              frame "Bad", Default {
              }
              frame "Idle" {
                n669 = Open VI Reference(type specifier VI Refnum (for type only)=refnum<vi> refnum ("类型说明符VI引用句柄（仅用于类型）"), vi path=w1066, options=128 ("选项")) -> (vi reference=w1067:refnum<vi>, error out=w1062:errorcluster)  [unwired: 3 in]
                n670 = call-by-ref "开始异步调用"(reference=w1067, error in=w1062, "CODMn量程切换"="CODMn量程选择", "总磷量程切换"="总磷量程选择", "总氮量程切换"="总氮量程选择", "氨氮量程切换"="氨氮量程选择", "参数"=w1065) -> (reference out=w1064:refnum<vi>, error out=w1063:errorcluster)  [unwired: 7 in]
                n671 = Close Reference(reference=w1064, error in (no error)=w1063) -> ()  [unwired: 1 out]
              }
            }
          }
        }
      }
      event "报警清除": Value Change {
        w1074 = FALSE ("氨氮中断报警")
        n672 = event-data() -> ()  [unwired: 1 in, 6 out]
        n673 = local read "氨氮、总磷模块"() -> (w1084:bool)
        n674 = local read "氨氮、总磷模块"() -> (w1075:bool)
        n675 = case shown="真" w1084 {
          tunnel: [errorcluster {"status"=FALSE, "code"=0, "source"=""} ("error out") w1127] -> w1081
          frame False {
          }
          frame True {
            n676 = call "多个线圈写入.vi"("values"=bool[] [TRUE], "starting address"=u16 2106, "Slave ID"=u8 1) -> ("error out"=w1127:errorcluster)  [unwired: 8 in]
          }
        }
        n677 = local read "总氮模块选择"() -> (w1083:bool)
        n678 = local read "总氮模块选择"() -> (w1076:bool)
        n679 = case shown="真" w1083 {
          tunnel: w1081 -> [w1120 w1123]
          tunnel: [w1120 w1121] -> w1080
          frame False {
          }
          frame True {
            n680 = call "多个线圈写入.vi"("Error in"=w1123, "values"=bool[] [TRUE], "starting address"=u16 2106, "Slave ID"=u8 2) -> ("error out"=w1121:errorcluster)  [unwired: 7 in]
          }
        }
        n681 = local read "CODMn选择"() -> (w1082:bool)
        n682 = local read "CODMn选择"() -> (w1077:bool)
        n683 = case shown="真" w1082 {
          tunnel: w1080 -> [w1114 w1118]
          tunnel: [w1114 w1115] -> w1071
          frame False {
          }
          frame True {
            n684 = call "多个线圈写入.vi"("Error in"=w1118, "values"=bool[] [TRUE], "starting address"=u16 2106, "Slave ID"=u8 3) -> ("error out"=w1115:errorcluster)  [unwired: 7 in]
          }
        }
        n685 = global write "质控中断报警全局.vi" "CODMn中断报警"(w1074) -> ()
        n686 = global write "质控中断报警全局.vi" "氨氮中断报警"(w1074) -> ()
        n687 = global write "质控中断报警全局.vi" "CODCr中断报警"(w1074) -> ()
        n688 = global write "质控中断报警全局.vi" "总氮中断报警"(w1074) -> ()
        n689 = global write "质控中断报警全局.vi" "总磷中断报警"(w1074) -> ()
        n690 = local read "CODCr选择"() -> (w1072:bool)
        n691 = local read "CODCr选择"() -> (w1073:bool)
        n692 = case shown="真" w1072 {
          tunnel: w1071 -> [w1091 w1095]
          tunnel: [w1091 w1092] -> w1070
          frame False {
          }
          frame True {
            n693 = call "多个线圈写入.vi"("Error in"=w1095, "values"=bool[] [TRUE], "starting address"=u16 2106, "Slave ID"=u8 4) -> ("error out"=w1092:errorcluster)  [unwired: 7 in]
          }
        }
        n694 = case shown="假" w1075 {
          tunnel: [w1109 w1110] -> w1078
          tunnel: w1070 -> [w1109 _]
          frame False {
          }
          frame True {
            n695 = call "多个线圈写入.vi"("values"=bool[] [FALSE], "starting address"=u16 2106, "Slave ID"=u8 1) -> ("error out"=w1110:errorcluster)  [unwired: 8 in]
          }
        }
        n696 = case shown="真" w1076 {
          tunnel: w1078 -> [w1103 w1106]
          tunnel: [w1103 w1104] -> w1079
          frame False {
          }
          frame True {
            n697 = call "多个线圈写入.vi"("Error in"=w1106, "values"=bool[] [FALSE], "starting address"=u16 2106, "Slave ID"=u8 2) -> ("error out"=w1104:errorcluster)  [unwired: 7 in]
          }
        }
        n698 = case shown="真" w1077 {
          tunnel: w1079 -> [w1097 w1101]
          tunnel: [w1097 w1098] -> w1069
          frame False {
          }
          frame True {
            n699 = call "多个线圈写入.vi"("Error in"=w1101, "values"=bool[] [FALSE], "starting address"=u16 2106, "Slave ID"=u8 3) -> ("error out"=w1098:errorcluster)  [unwired: 7 in]
          }
        }
        n700 = case shown="真" w1073 {
          tunnel: w1069 -> [w1085 w1089]
          tunnel: [w1085 w1086] -> w1068
          frame False {
          }
          frame True {
            n701 = call "多个线圈写入.vi"("Error in"=w1089, "values"=bool[] [FALSE], "starting address"=u16 2106, "Slave ID"=u8 4) -> ("error out"=w1086:errorcluster)  [unwired: 7 in]
          }
        }
      }
      event "氨氮加标回收启动": Value Change {
        n702 = event-data() -> ()  [unwired: 1 in, 6 out]
        n703 = Two Button Dialog(message="确定启动氨氮的加标回收？" ("消息"), 1:"否" ("F按钮名称（“取消”）"), 2:"是" ("T按钮名称（“确定”）")) -> (T button?=w1131:bool)
        n704 = case shown="真" w1131 {
          frame False {
          }
          frame True {
            n705 = vi-ref "质控单元.lvlib:氨氮流程质控自动启动.vi"() -> (w1137:refnum<vi>)
            n706 = property class="VI"(reference=w1137) -> ("Name"=w1135:string, "Exec.State"=w1136:T16)  [unwired: 1 in, 2 out]
            n707 = case shown="\"Idle\"" w1136 {
              tunnel: w1135 -> [_ w1141 _ _]
              frame "Bad", Default {
              }
              frame "Idle" {
                n708 = local read "氨氮量程选择"() -> (w1140:enum32{"H", "L", "AUTO"})
                n709 = Open VI Reference(type specifier VI Refnum (for type only)=refnum<vi> refnum ("类型说明符VI引用句柄（仅用于类型）"), vi path=w1141, options=128 ("选项")) -> (vi reference=w1145:refnum<vi>, error out=w1139:errorcluster)  [unwired: 3 in]
                n710 = call-by-ref "开始异步调用"(reference=w1145, error in=w1139, "氨氮量程切换"=w1140) -> (reference out=w1144:refnum<vi>, error out=w1138:errorcluster)  [unwired: 11 in]
                n711 = Close Reference(reference=w1144, error in (no error)=w1138) -> ()  [unwired: 1 out]
              }
              frame "Run top level" {
              }
              frame "Running" {
              }
            }
          }
        }
      }
      event "总磷总氮加标回收启动": Value Change {
        w1148 = TRUE ("总氮")
        w1149 = FALSE ("氨氮")
        n712 = event-data() -> ()  [unwired: 1 in, 6 out]
        n713 = call "质控启动参数选择对话框.vi"("COD"=w1149, "总氮"=w1148, "总磷"=w1148, "氨氮"=w1149) -> ("确定启动"=w1147:bool, "启动模块"=w1146:T3)  [unwired: 5 in, 1 out]
        n714 = case shown="真" w1147 {
          tunnel: w1146 -> [_ w1152]
          frame False {
          }
          frame True {
            n715 = vi-ref "质控单元.lvlib:总磷总氮流程质控自动启动.vi"() -> (w1155:refnum<vi>)
            n716 = Unbundle By Name(w1152) -> ("总磷"=w1151:bool, "总氮"=w1150:bool)
            n717 = property class="VI"(reference=w1155) -> ("Name"=w1153:string, "Exec.State"=w1154:T16)  [unwired: 1 in, 2 out]
            n718 = case shown="\"Idle\"" w1154 {
              tunnel: w1153 -> [_ w1164 _ _]
              tunnel: w1151 -> [_ w1157 _ _]
              tunnel: w1150 -> [_ w1156 _ _]
              frame "Bad", Default {
              }
              frame "Idle" {
                n719 = Bundle By Name(cluster=T14 {"是否启用仪器"=FALSE, "CODMn"={"启动测量模式"={"测量模式"=enum."水样测量"}, "确定按钮"=FALSE}, "启动模块"={"氨氮"=FALSE, "总磷"=FALSE, "总氮"=FALSE, "COD"=FALSE}, "常规启动"=FALSE, "直接启动"=FALSE} ("参数"), "启动模块.总磷"=w1157, "启动模块.总氮"=w1156) -> (w1158:T14)
                n720 = local read "总氮量程选择"() -> (w1161:enum32{"H", "L", "AUTO"})
                n721 = local read "总磷量程选择"() -> (w1160:enum32{"H", "L", "AUTO"})
                n722 = Open VI Reference(type specifier VI Refnum (for type only)=refnum<vi> refnum ("类型说明符VI引用句柄（仅用于类型）"), vi path=w1164, options=128 ("选项")) -> (vi reference=w1168:refnum<vi>, error out=w1162:errorcluster)  [unwired: 3 in]
                n723 = call-by-ref "开始异步调用"(reference=w1168, error in=w1162, "总磷量程切换"=w1160, "总氮量程切换"=w1161, "参数"=w1158) -> (reference out=w1167:refnum<vi>, error out=w1163:errorcluster)  [unwired: 9 in]
                n724 = Close Reference(reference=w1167, error in (no error)=w1163) -> ()  [unwired: 1 out]
              }
              frame "Run top level" {
              }
              frame "Running" {
              }
            }
          }
        }
      }
      event "CODMn加标回收启动": Value Change {
        n725 = event-data() -> ()  [unwired: 1 in, 6 out]
        n726 = Two Button Dialog(message="确定启动CODMn的加标回收？" ("消息"), 1:"否" ("F按钮名称（“取消”）"), 2:"是" ("T按钮名称（“确定”）")) -> (T button?=w1169:bool)
        n727 = case shown="真" w1169 {
          frame False {
          }
          frame True {
            n728 = vi-ref "CODMn流程质控自动启动.vi"() -> (w1175:refnum<vi>)
            n729 = property class="VI"(reference=w1175) -> ("Name"=w1173:string, "Exec.State"=w1174:T16)  [unwired: 1 in, 2 out]
            n730 = case shown="\"Idle\"" w1174 {
              tunnel: w1173 -> [_ w1179 _ _]
              frame "Bad", Default {
              }
              frame "Idle" {
                n731 = local read "CODMn量程选择"() -> (w1176:enum32{"H", "L", "AUTO"})
                n732 = Open VI Reference(type specifier VI Refnum (for type only)=refnum<vi> refnum ("类型说明符VI引用句柄（仅用于类型）"), vi path=w1179, options=128 ("选项")) -> (vi reference=w1183:refnum<vi>, error out=w1178:errorcluster)  [unwired: 3 in]
                n733 = call-by-ref "开始异步调用"(reference=w1183, error in=w1178, "CODMn量程切换"=w1176) -> (reference out=w1182:refnum<vi>, error out=w1177:errorcluster)  [unwired: 10 in]
                n734 = Close Reference(reference=w1182, error in (no error)=w1177) -> ()  [unwired: 1 out]
              }
              frame "Run top level" {
              }
              frame "Running" {
              }
            }
          }
        }
      }
      event "CODCr加标回收启动": Value Change {
        n735 = event-data() -> ()  [unwired: 1 in, 6 out]
        n736 = Two Button Dialog(message="确定启动CODCr的加标回收？" ("消息"), 1:"否" ("F按钮名称（“取消”）"), 2:"是" ("T按钮名称（“确定”）")) -> (T button?=w1184:bool)
        n737 = case shown="真" w1184 {
          frame False {
          }
          frame True {
            n738 = vi-ref "CODCr流程质控自动启动.vi"() -> (w1190:refnum<vi>)
            n739 = property class="VI"(reference=w1190) -> ("Name"=w1188:string, "Exec.State"=w1189:T16)  [unwired: 1 in, 2 out]
            n740 = case shown="\"Idle\"" w1189 {
              tunnel: w1188 -> [_ w1194 _ _]
              frame "Bad", Default {
              }
              frame "Idle" {
                n741 = local read "CODCr量程选择"() -> (w1191:enum32{"H", "L", "AUTO"})
                n742 = Open VI Reference(type specifier VI Refnum (for type only)=refnum<vi> refnum ("类型说明符VI引用句柄（仅用于类型）"), vi path=w1194, options=128 ("选项")) -> (vi reference=w1198:refnum<vi>, error out=w1193:errorcluster)  [unwired: 3 in]
                n743 = call-by-ref "开始异步调用"(reference=w1198, error in=w1193, "CODMn量程切换"=w1191) -> (reference out=w1197:refnum<vi>, error out=w1192:errorcluster)  [unwired: 10 in]
                n744 = Close Reference(reference=w1197, error in (no error)=w1192) -> ()  [unwired: 1 out]
              }
              frame "Run top level" {
              }
              frame "Running" {
              }
            }
          }
        }
      }
      event "平行样测试": Value Change {
        n745 = event-data() -> ()  [unwired: 1 in, 6 out]
        n746 = flat-sequence {
          tunnel: [w1204] -> w1202
          tunnel: [w1206] -> w1201
          tunnel: [w1205] -> w1200
          tunnel: w1199 -> [w1203]
          tunnel: w1202 -> [w1213]
          tunnel: w1201 -> [w1212]
          tunnel: w1200 -> [w1211]
          frame #0 {
            n747 = Cancel Notification(0:w1203) -> ()  [unwired: 1 in, 3 out]
            n748 = call "平行样启动流程对话框.vi"() -> ("启动模块"=w1204:cluster{"氨氮1":bool, "总磷1":bool, " COD1":bool}, "直接启动"=w1205:bool, "常规启动"=w1206:bool)  [unwired: 8 in, 1 out]
            "常规启动 2" <- w1206
            "直接启动 2" <- w1205
            "启动模块 2" <- w1204
          }
          frame #1 {
            n749 = Bundle By Name(cluster=T5 {"是否启用仪器"=FALSE, "CODMn"={"启动测量模式"={"测量模式"=enum."水样测量"}, "确定按钮"=TRUE}, "启动模块"={"氨氮1"=FALSE, "总磷1"=FALSE, " COD1"=FALSE}, "常规启动"=FALSE, "直接启动"=FALSE} ("参数"), "是否启用仪器"=TRUE, "启动模块"=w1213, "常规启动"=w1212, "直接启动"=w1211) -> (w1208:T5)
            "输出簇 2" <- w1208
            n750 = vi-ref "一体站流程平行样自动启动.vi"() -> (w1209:refnum<vi>)
            n751 = property class="VI"(reference=w1209) -> ("Name"=w1210:string, "Exec.State"=w1207:T16)  [unwired: 1 in, 2 out]
            n752 = case shown="\"Idle\"" w1207 {
              tunnel: w1210 -> [_ w1222]
              tunnel: w1208 -> [_ w1216]
              frame "Bad", Default {
              }
              frame "Idle" {
                n753 = Open VI Reference(type specifier VI Refnum (for type only)=refnum<vi> refnum ("类型说明符VI引用句柄（仅用于类型）"), vi path=w1222, options=128 ("选项")) -> (vi reference=w1223:refnum<vi>, error out=w1221:errorcluster)  [unwired: 3 in]
                n754 = call-by-ref "开始异步调用"(reference=w1223, error in=w1221, "参数"=w1216) -> (reference out=w1218:refnum<vi>, error out=w1217:errorcluster)  [unwired: 9 in]
                n755 = Close Reference(reference=w1218, error in (no error)=w1217) -> ()  [unwired: 1 out]
              }
            }
          }
        }
      }
      event "停止测量": Value Change {
        w1224 = TRUE ("氨氮")
        # "停止采配水、氨氮、总磷总氮、COD、质控"
        n756 = event-data() -> ()  [unwired: 1 in, 6 out]
        n757 = call "质控启动参数选择对话框.vi"("COD"=w1224, "总氮"=w1224, "总磷"=w1224, "氨氮"=w1224) -> ("确定启动"=w1225:bool, "启动模块"=w1226:T3)  [unwired: 5 in, 1 out]
        n758 = case shown="真" w1225 {
          tunnel: w1226 -> [_ w1236]
          frame False {
          }
          frame True {
            n759 = Unbundle By Name(w1236) -> ("氨氮"=w1234:bool, "总磷"=w1233:bool, "总氮"=w1232:bool, "COD"=w1235:bool)
            n760 = Or(x=w1233, y=w1232) -> (x .or. y?=w1231:bool)
            n761 = case shown="真" w1235 {
              frame False {
              }
              frame True {
                n762 = call "CODMn停止命令 (子VI).vi"() -> ()  [unwired: 12 in]
                n763 = Obtain Notifier(name (unnamed)="CODMn" ("名称（未命名）"), notification data type=FALSE) -> (notifier out=w1262:refnum<notifier>)  [unwired: 2 in, 2 out]
                n764 = Send Notification(notification=TRUE ("通知"), notifier=w1262) -> ()  [unwired: 1 in, 2 out]
                n765 = call "单个写入.vi"("value"=u16 2, "address"=u16 103, "Slave ID"=u8 3) -> ()  [unwired: 8 in, 1 out]
              }
            }
            n766 = case shown="真" w1234 {
              frame False {
              }
              frame True {
                n767 = Obtain Queue(name (unnamed)="NH3N" ("名称（未命名）"), element data type=cluster{"命令":string, "data":variant} {"命令"="", "data"=variant}) -> (queue out=w1258:refnum<queue>)  [unwired: 3 in, 2 out]
                n768 = Enqueue Element(queue=w1258, element=cluster{"命令":string, "data":variant} {"命令"="启动", "data"=variant(cluster{"站号":u16, "控制命令输出":u16[]} {"站号"=1, "控制命令输出"=[2816]})} ("元素")) -> ()  [unwired: 2 in, 3 out]
                n769 = Obtain Notifier(name (unnamed)="NH3N" ("名称（未命名）"), notification data type=FALSE) -> (notifier out=w1254:refnum<notifier>)  [unwired: 2 in, 2 out]
                n770 = Send Notification(notification=TRUE ("通知"), notifier=w1254) -> ()  [unwired: 1 in, 2 out]
                n771 = call "单个写入.vi"("value"=u16 2, "address"=u16 103, "Slave ID"=u8 1) -> ()  [unwired: 8 in, 1 out]
              }
            }
            n772 = case shown="真" w1231 {
              frame False {
              }
              frame True {
                n773 = Obtain Queue(name (unnamed)="TP" ("名称（未命名）"), element data type=cluster{"命令":string, "data":variant} {"命令"="", "data"=variant}) -> (queue out=w1247:refnum<queue>)  [unwired: 3 in, 2 out]
                n774 = Enqueue Element(queue=w1247, element=cluster{"命令":string, "data":variant} {"命令"="启动", "data"=variant(cluster{"站号":u16, "控制命令输出":u16[]} {"站号"=1, "控制命令输出"=[2816]})} ("元素")) -> ()  [unwired: 2 in, 3 out]
                n775 = Obtain Notifier(name (unnamed)="TNTP" ("名称（未命名）"), notification data type=FALSE) -> (notifier out=w1243:refnum<notifier>)  [unwired: 2 in, 2 out]
                n776 = Send Notification(notification=TRUE ("通知"), notifier=w1243) -> ()  [unwired: 1 in, 2 out]
                n777 = call "单个写入.vi"("value"=u16 2, "address"=u16 103, "Slave ID"=u8 2) -> ()  [unwired: 8 in, 1 out]
              }
            }
          }
        }
        n778 = Send Notification(notification=TRUE ("通知"), notifier=w1230) -> ()  [unwired: 1 in, 2 out]
        n779 = Enqueue Element At Opposite End(queue=w1227, element=T15 {"命令"="单个写入", {"starting address"=300, "holding register value"=2}} ("元素")) -> ()  [unwired: 2 in, 3 out]
      }
      event "查看": Value Change {
        n780 = event-data() -> ()  [unwired: 1 in, 6 out]
        n781 = property on="窗格" class="Pane"("Origin"=T7 {"Horizontal"=0, "Vertical"=600} ("原点")) -> ()  [unwired: 2 in, 2 out]
      }
      event "返回": Value Change {
        n782 = event-data() -> ()  [unwired: 1 in, 6 out]
        n783 = property on="窗格" class="Pane"("Origin"=T7 {"Horizontal"=0, "Vertical"=0} ("原点")) -> ()  [unwired: 2 in, 2 out]
      }
    }
  }
  n784 = call "质控参数读取.vi"("section"="CODCr质控参数", "error in (no error)"=w18) -> ("参数"=w19:T8)  [unwired: 8 in, 1 out]
  n785 = Unbundle By Name(w19) -> ("量程"=→"CODCr量程":dbl, "检出限"=→"CODCr检出限":dbl, "加标前水样浓度"=→"CODCr加标前水样浓度":dbl, "加标后水样浓度"=→"CODCr加标后水样浓度":dbl, "加标水杯定容体积"=→"CODCr加标水杯定容体积":dbl, "加标母液浓度"=→"CODCr母液浓度":dbl, "加标体积"=→"CODCr加标体积":dbl, "加标回收率"=→"CODCr加标回收率":dbl)
  n786 = call-dynamic "Close Session.vi"("error in (no error)"=w53, "MB_Serial session"=w23) -> ()  [unwired: 9 in, 1 out]
  "VISA Resource" <- w22
  "Serial Config" <- w21
